vi "DialogRenameVI.vi"(0 "ObjectIn":refnum<class "ClassWriterNative.lvclass">, 1 "ProjectItem":refnum<vi>, 5 "error in (no error)":errorcluster) -> (14 "ObjectOut":refnum<class "ClassWriterNative.lvclass">, 15 "Cancelled":bool, 16 "RenameOption":T1, 19 "error out":errorcluster)   [LabVIEW 2020, in "ClassWriterNative.lvclass"]
uses:
  <resource>/Framework/Providers/Open_GDS/ClassProviders/Provider_LvNativeClass/ClassWriterNative_class/ClassWriterNative.lvclass
  <resource>/Framework/Providers/Open_GDS/ClassProviders/Common/LvIcon_class/GDSLvIcon_ColorControl.ctl
  <resource>/Framework/Providers/Open_GDS/ClassProviders/Provider_BaseClassInterface/ClassWriter_class/RenameViOption.ctl
  <vilib>/Utility/miscctls.llb/LVPoint32TypeDef.ctl
  <vilib>/picture/picture.llb/imagedata.ctl
  <resource>/Framework/Providers/Open_GDS/ClassProviders/Common/LvIcon_class/subvis/GDSLvIcon_TextDataType.ctl
  <resource>/Framework/Providers/Open_GDS/ClassProviders/Common/LvIcon_class/GDSLvIcon_WordCompressionType.ctl
  <resource>/Framework/Providers/Open_GDS/ClassProviders/Common/LvIcon_class/GDSLvIcon_TextAlignment.ctl
  <vilib>/Utility/miscctls.llb/LVPositionTypeDef.ctl
  <vilib>/Utility/miscctls.llb/LVPointTypeDef.ctl
  <resource>/Framework/Providers/Open_GDS/ClassProviders/Provider_BaseClassInterface/ClassWriter_class/ClassWriter.lvclass
panel:
  in  "_ShowContextHelp":bool
  in  "Help":bool
  out "ProductPicture":picture
  out "Ballon":cluster{"Text":string}
  in  "_MethodIcons":bool
  out "_IconPreview":picture caption="Icon Preview"
  in  "_Cancel":bool
  in  "_RenameVI":bool
  out "DragIcon":picture
  in  "FloodFillMask":bool
  in  "_IconSearchText":string caption="Icon search text"
  in  "_Manage":bool
  in  "_Folders":u16(ring) caption="Folders" items=["<All icons>", "...ikael\\Documents\\LabVIEW Data\\Glyphs", "...\\resource\\Framework\\Providers\\Icons", "...Framework\\Providers\\Open_GDS\\Glyphs", "...\\Framework\\Providers\\Open_GDS\\Icons"]
  out "Icons":picture
  in  "_HideHeader":bool=TRUE caption="Force Capital Letters"
  in  "_IconSize":u16(ring) caption="Icon Size" items=["Full", "1 c-term high", "2 c-term high", "3 c-term high"]
  out "Tree":string[](tree)
  in  "_TextAlignment":u16(ring) caption="Text Alignment" items=["Center", "Left", "Right"]
  in  "_MethodIconName":string caption="Body Text"
  in  "_BodyBk":T2 caption="Body Background"
  in  "_BodyText":T2 caption="Body text"
  in  "_FontCompression":enum16{"Auto", "On", "Off"}(ring) caption="Font Compression"
  in  "_CapitalOnly":bool=TRUE caption="Force Capital Letters"
  out "_After":picture caption="New"
  out "_Before":picture caption="Current"
  out "_VIPath":path caption="VI Path"
  in  "NewName":string caption="New Name"
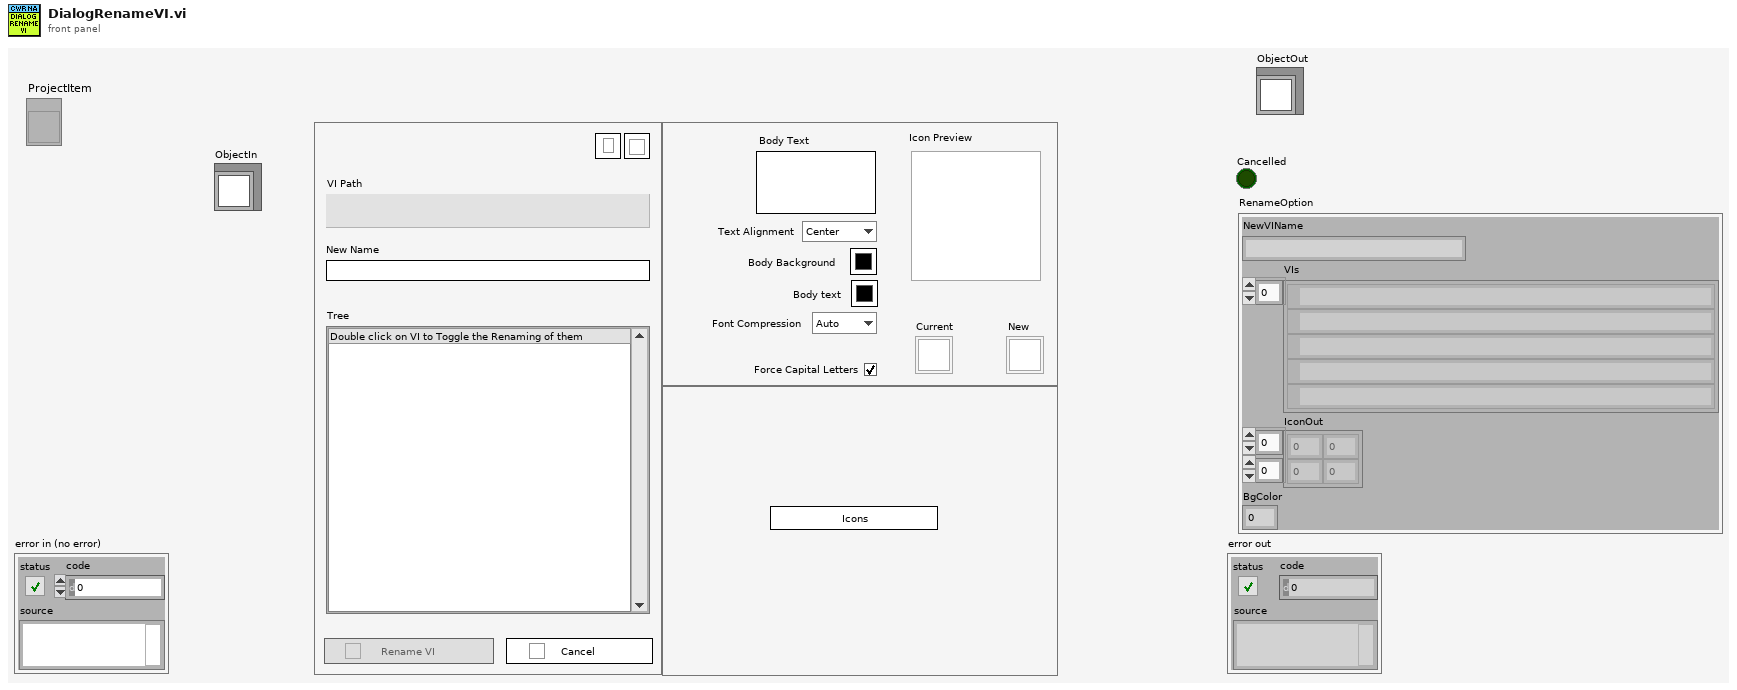
[diagram p1: front panel]
types:
  T1 = typedef "ClassWriter.lvclass/RenameViOption.ctl" = cluster{"NewVIName":string, "VIs":path[], "IconOut":u8[][], "BgColor":u8}
  T2 = typedef "GDSLvIcon_ColorControl.ctl" = cluster{"Decal":bool, "Color":u32}
  T3 = typedef "LVPoint32TypeDef.ctl" = cluster{"Horizontal":i32, "Vertical":i32}
  T4 = typedef "imagedata.ctl" = cluster{"image type":i32, "image depth":i32, "image":u8[], "mask":u8[], "colors":u32[], "Rectangle":cluster{"left":i16, "top":i16, "right":i16, "bottom":i16}}
  T5 = cluster{"ClassIndex":i32, "NewName":string, "Cancelled":bool, "VIref":refnum<vi>, "Class":refnum<vi>, "ClassPath":path, "VIPath":path, "Classes":cluster{i32, refnum<vi>, cluster{"Path":path, "Name":string, "QualifiedName":string}[]}[], "ClassInfos":cluster{"ClassName":string, "ViRelPath":path, "AllVIs":string[], "VI-Path":path, "Private":bool}[], "TreeTags":string[], "Selected":i32[], "CurrentIcon":cluster{"BgIcon":u8[][], "BgIconOffset":cluster{"X":i32, "Y":i32}, "BgIconMask":u8[], "ColorsOkayforiconToBeOnTopOf":u8[]}, "StartIconSize":u16, "Offset":cluster{"X":i32, "Y":i32}, "OldOffset":cluster{"X":i32, "Y":i32}, "ConnectorPaneHeight":i32[], "BodyIcon":u8[][], "Icon exist":bool, "HeaderIcon":u8[][], "BodyIconWidth":i32, "BodyIconHeight":i32, "Frame thickness":i32, "StartRow":i32, "FrameColor":u32, "TextBounds":cluster{"FirstRow":i32, "FirstColumn":i32, "LastRow":i32, "LastColumn":i32}, "Header exists":bool, "HeaderBkColor":u32, "DraggingIcon":bool, "DraggingText":bool, "StartTextDraggingPos":T3, "IconSelected":i32, "BgIconOffset":cluster{"X":i32, "Y":i32}, "IconDropped":i32, "Moving":bool, "Folders":path[], "Icons":T4[], "IconPos":cluster{"left":i16, "top":i16, "right":i16, "bottom":i16}[], "IconPaths":cluster{i32, "path out":path}[], "IconNames":string[], "BgIcon":u8[][], "BgIconMask":u8[], "RenameOption":cluster{"NewVIName":string, "VIs":path[], "IconOut":u8[][], "BgColor":u8}, "StartTime":i32, "FileExtension":string}
  T6 = cluster{"Child Text":string[], "Child Tag":string, "Item Indent":i32, "Child Only?":bool, "Glyph Index":i32}[]
  T7 = cluster{"ClassName":string, "ViRelPath":path, "AllVIs":string[], "VI-Path":path, "Private":bool}
  T8 = enum32{"invalid scope", "public", "private", "protected", "community"}
  T9 = enum8{"Enabled", "Disabled", "Disabled and Grayed Out"}
  T10 = typedef "GDSLvIcon_TextDataType.ctl" = cluster{"Text":string, "Allow Only Capital Chars":bool, "Compression":T11, "Alignment":T12}
  T11 = typedef "GDSLvIcon_WordCompressionType.ctl" = enum16{"Auto", "On", "Off"}
  T12 = typedef "GDSLvIcon_TextAlignment.ctl" = enum16{"Center", "Left", "Right"}
  T13 = typedef "LVPositionTypeDef.ctl" = cluster{"Left":i32, "Top":i32}
  T14 = typedef "LVPointTypeDef.ctl" = cluster{"Horizontal":i16, "Vertical":i16}
  T15 = cluster{"Path":path, "Name":string, "QualifiedName":string}
  T16 = cluster{i32, refnum<vi>, cluster{"Path":path, "Name":string, "QualifiedName":string}[]}
  T17 = cluster{i32, refnum<vi>, cluster{"Path":path, "Name":string, "QualifiedName":string}[]}[]
  T18 = cluster{"Path":path, "Name":string, "QualifiedName":string}[]
  T19 = cluster{"ClassName":string, "ViRelPath":path, "AllVIs":string[], "VI-Path":path, "Private":bool}[]
  T20 = cluster{"BgIcon":u8[][], "BgIconOffset":cluster{"X":i32, "Y":i32}, "BgIconMask":u8[], "ColorsOkayforiconToBeOnTopOf":u8[]}
  T21 = cluster{"FirstRow":i32, "FirstColumn":i32, "LastRow":i32, "LastColumn":i32}
  T22 = typedef "LVBoundsTypeDef.ctl" = cluster{"Width":u32, "Height":u32}
  T23 = cluster{"left":i16, "top":i16, "right":i16, "bottom":i16}[]
  T24 = typedef "eventvkey.ctl" = enum16{"ASCII", "Enter", "Return", "Shift", "Ctrl", "Alt", "Cmd", "Opt", "Caps", "NumLock", "Clear", "Break", "Up", "Down", "Left", "Right", "Insert", "Delete", "Home", "End", "PageUp", "PageDown", "Escape", "Help", "Pause", "ScrollLock", "F1", "F2", "F3", "F4", "F5", "F6", "F7", "F8", "F9", "F10", "F11", "F12", "F13", "F14", "F15", "F16", "F17", "F18", "F19", "F20", "F21", "F22", "F23", "F24", "Play", "VolumeUp", "VolumeDown", "Mute", "Two Byte Char"}
  T25 = cluster{"Shift":bool, "Ctrl":bool, "Alt":bool, "Cmd":bool, "Opt":bool}
  T26 = typedef "LVMouseTypeDef.ctl" = cluster{"Mouse Position":cluster{"X":i32, "Y":i32}, "Mouse Modifiers":cluster{"Button Down":bool, "Shift Mod":bool, "Menu Mod":bool, "Option Mod":bool}}
  T27 = cluster{"left":i16, "top":i16, "right":i16, "bottom":i16}
  T28 = cluster{"NewVIName":string, "VIs":path[], "IconOut":u8[][], "BgColor":u8}
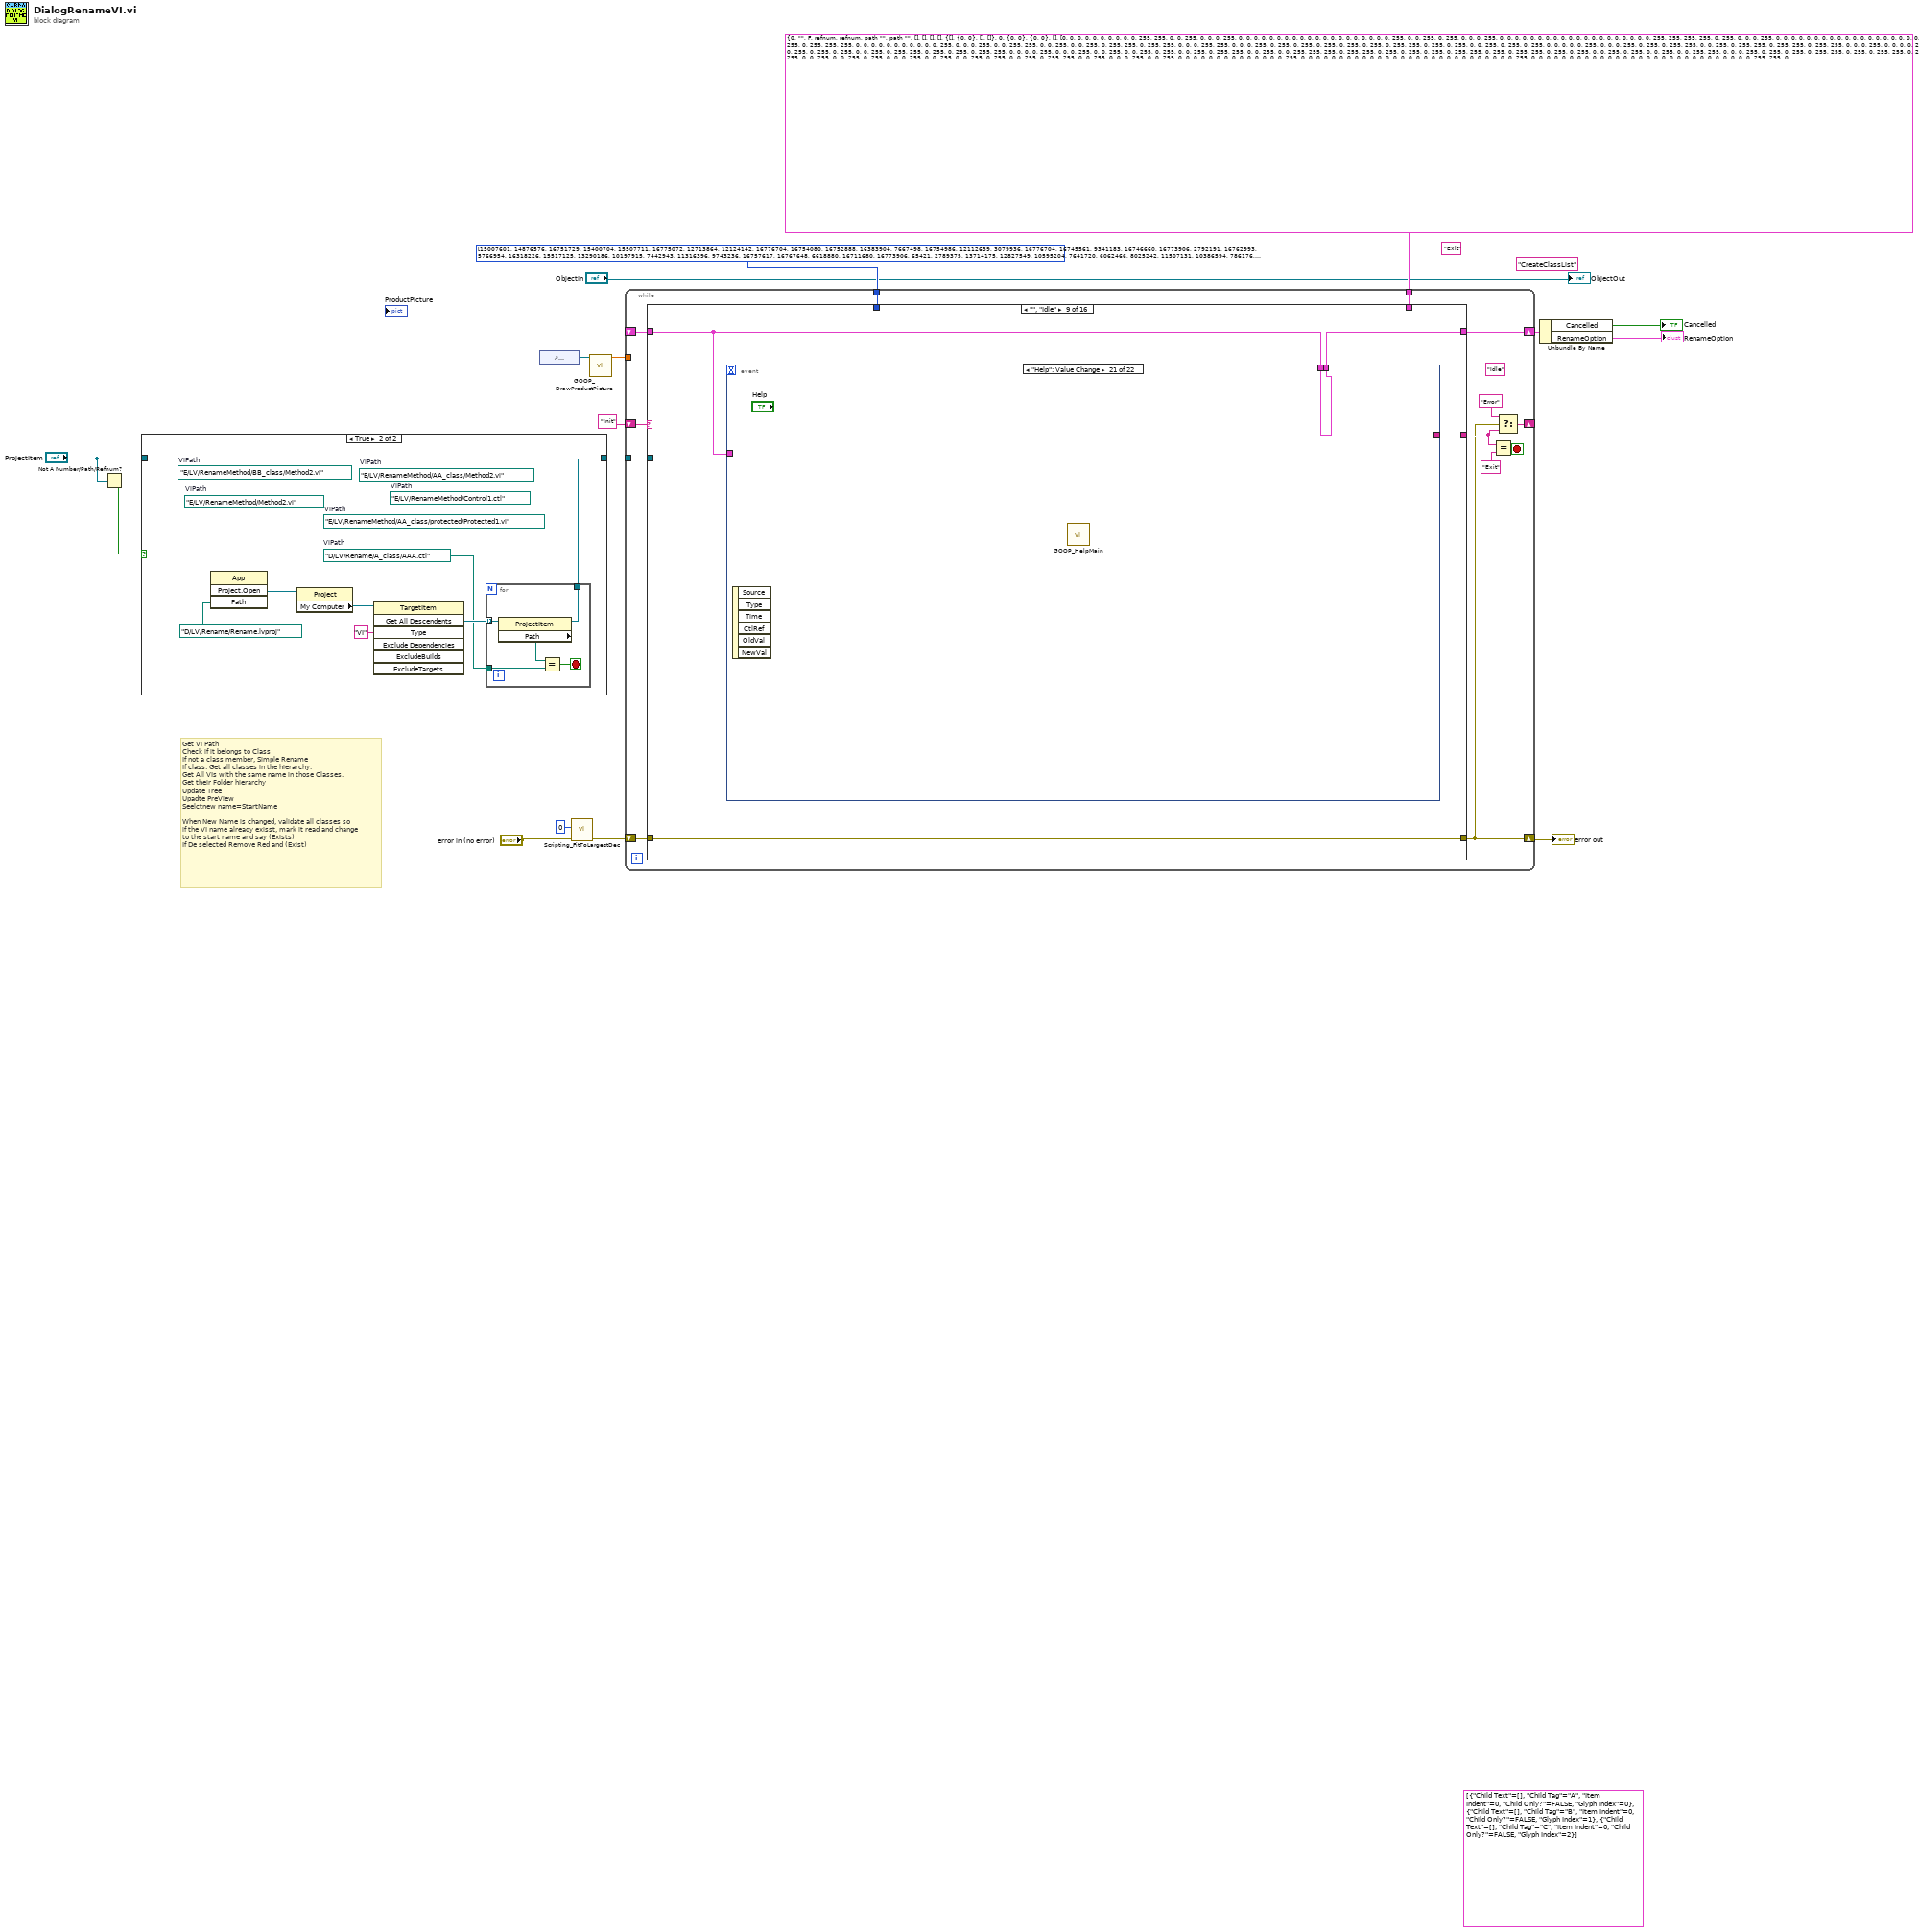
[diagram p0: block diagram]
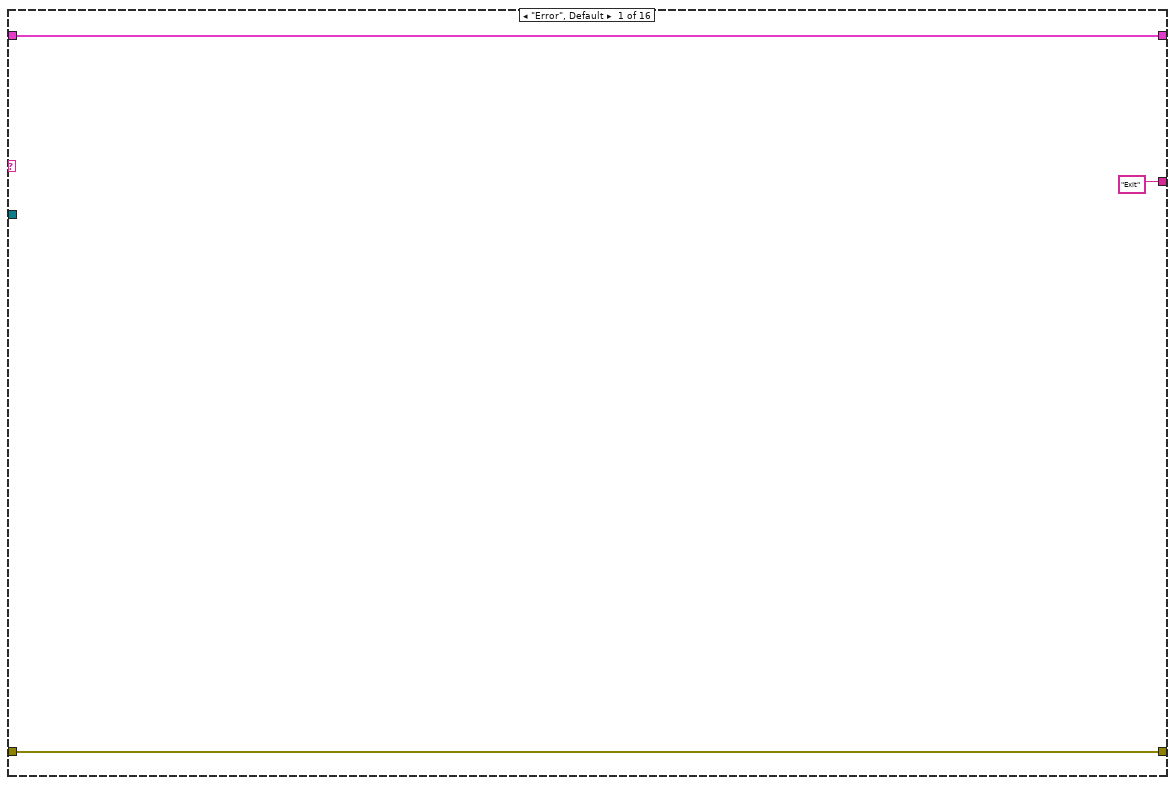
[diagram p3: hidden frame]
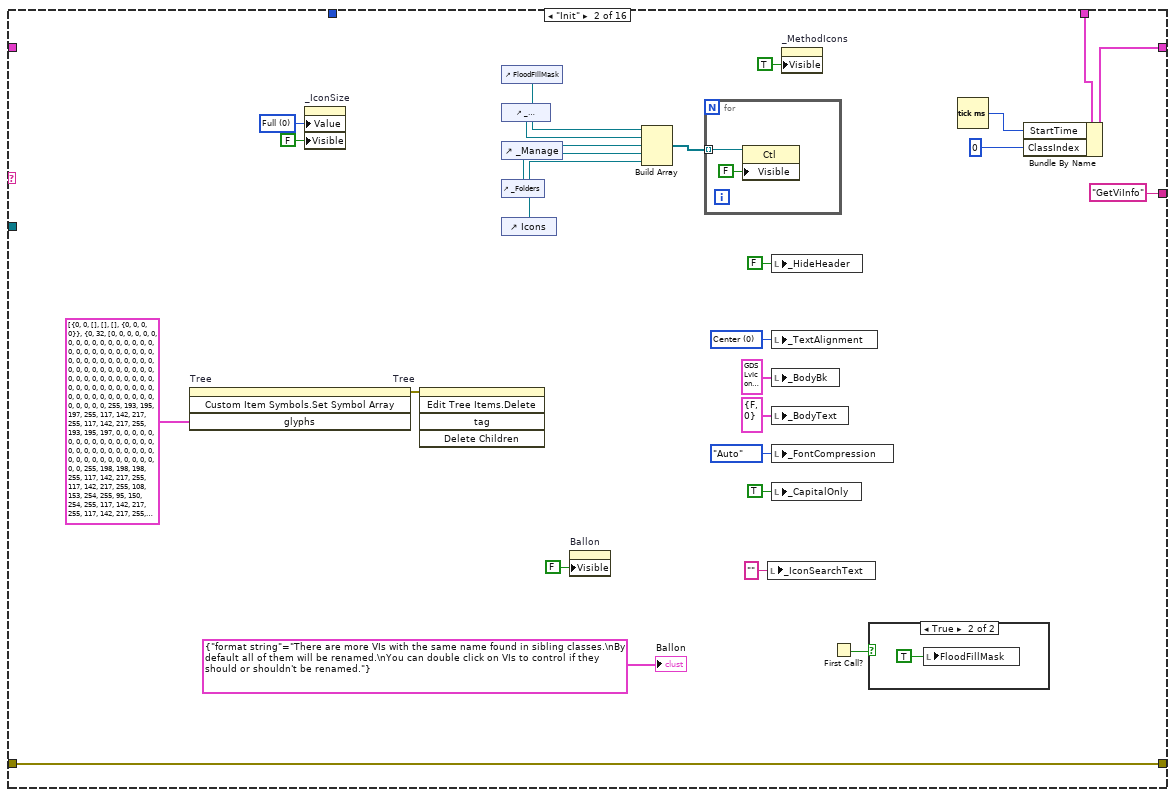
[diagram p4: hidden frame]
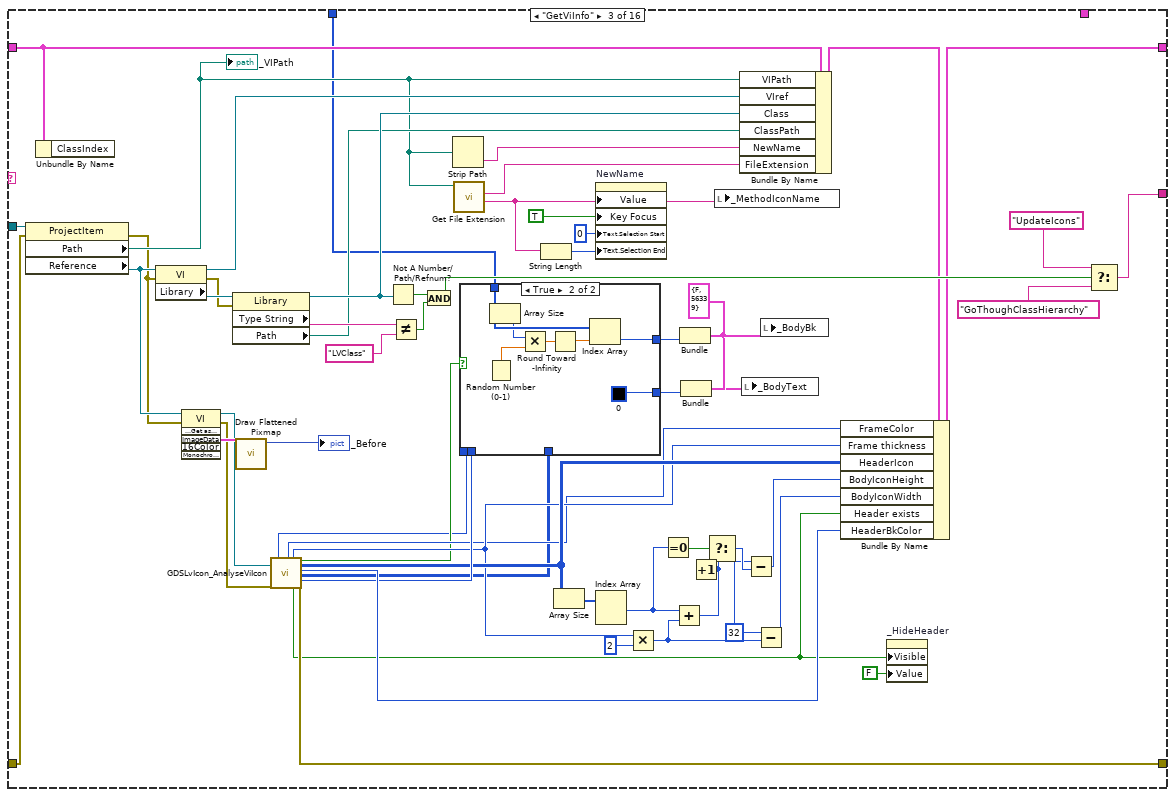
[diagram p6: hidden frame]
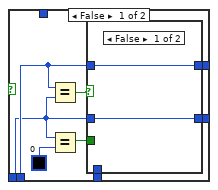
[diagram p7: hidden frame]
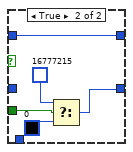
[diagram p8: hidden frame]
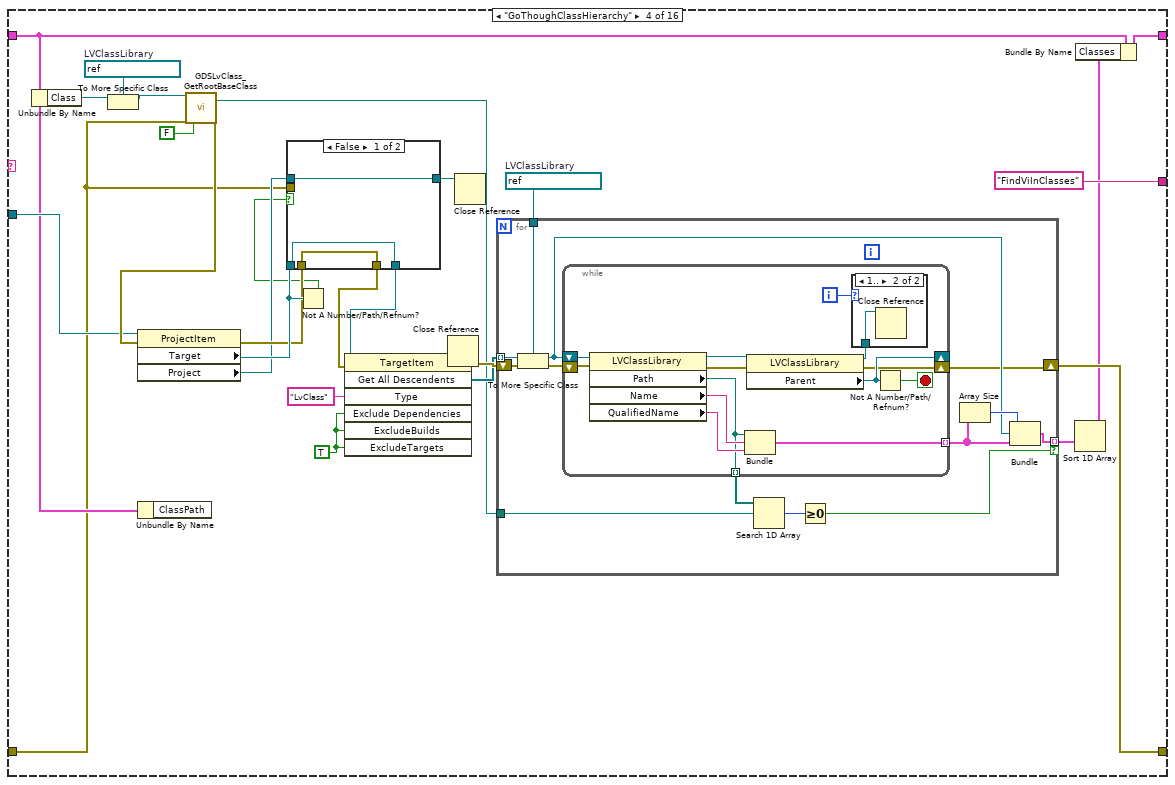
[diagram p9: hidden frame]
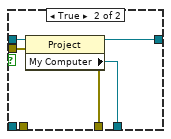
[diagram p10: hidden frame]
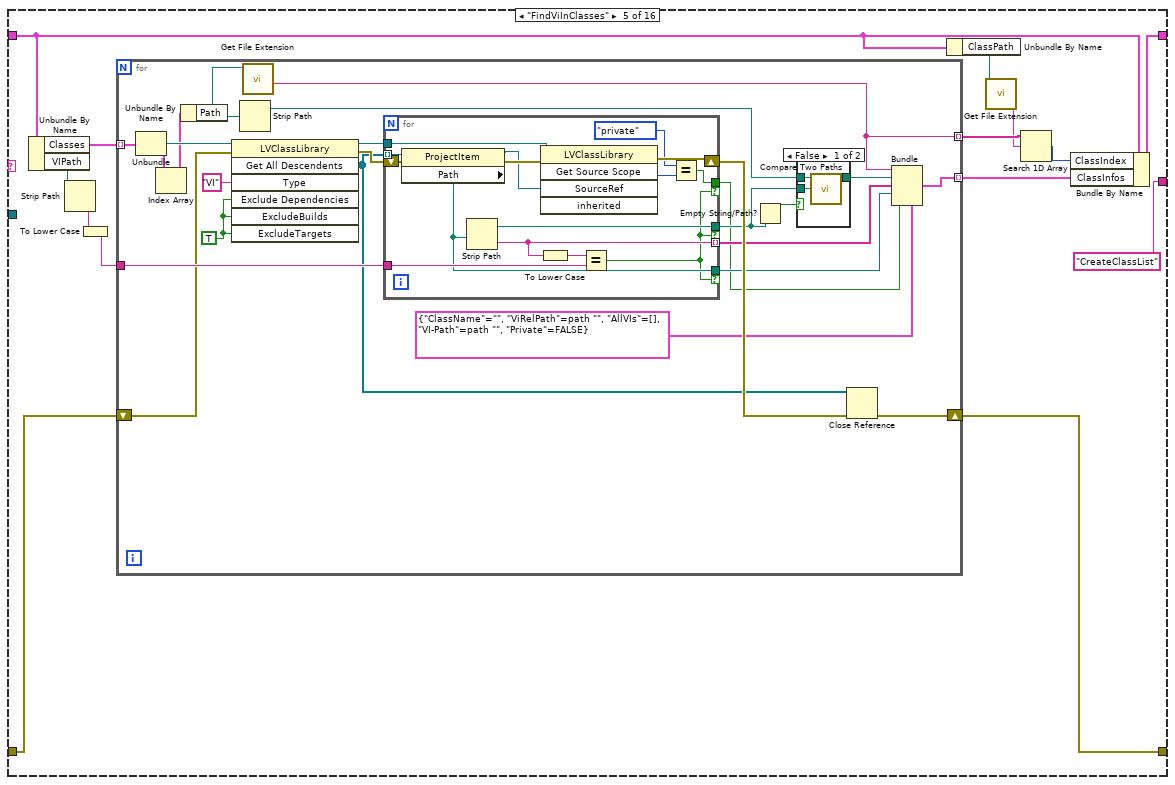
[diagram p12: hidden frame]
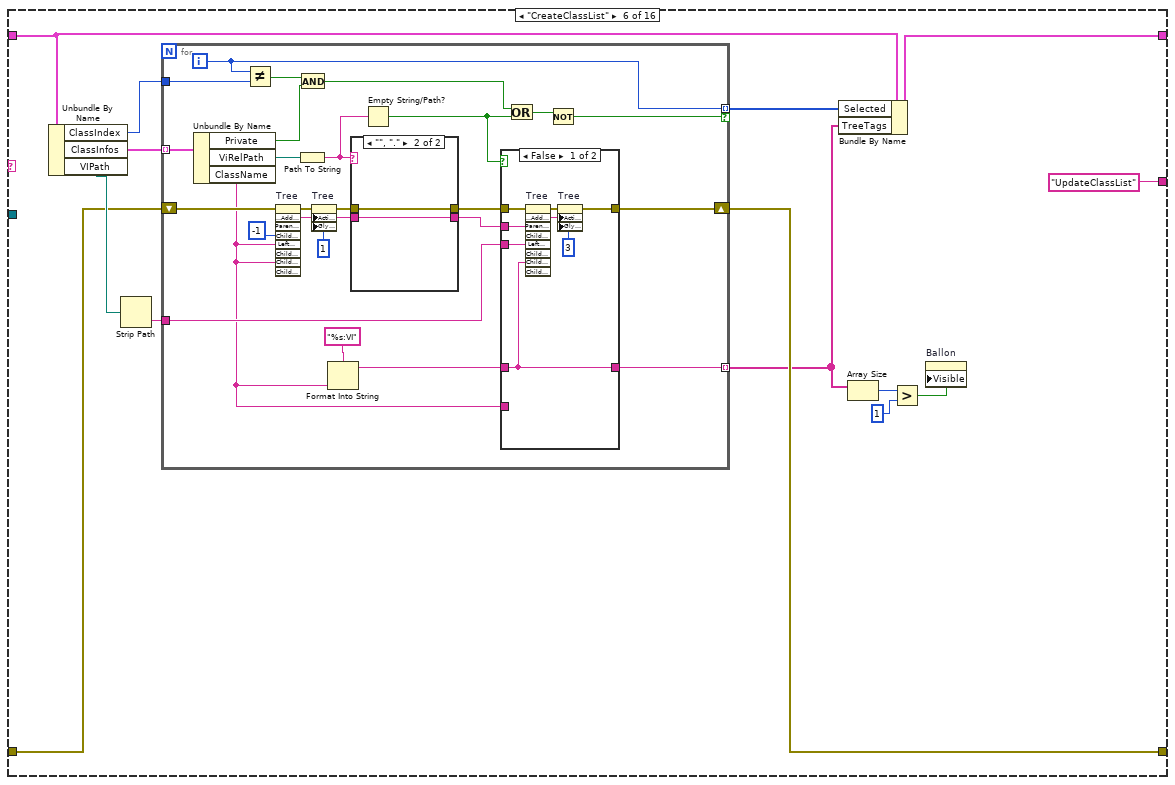
[diagram p14: hidden frame]
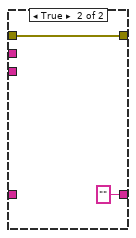
[diagram p15: hidden frame]
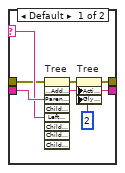
[diagram p16: hidden frame]
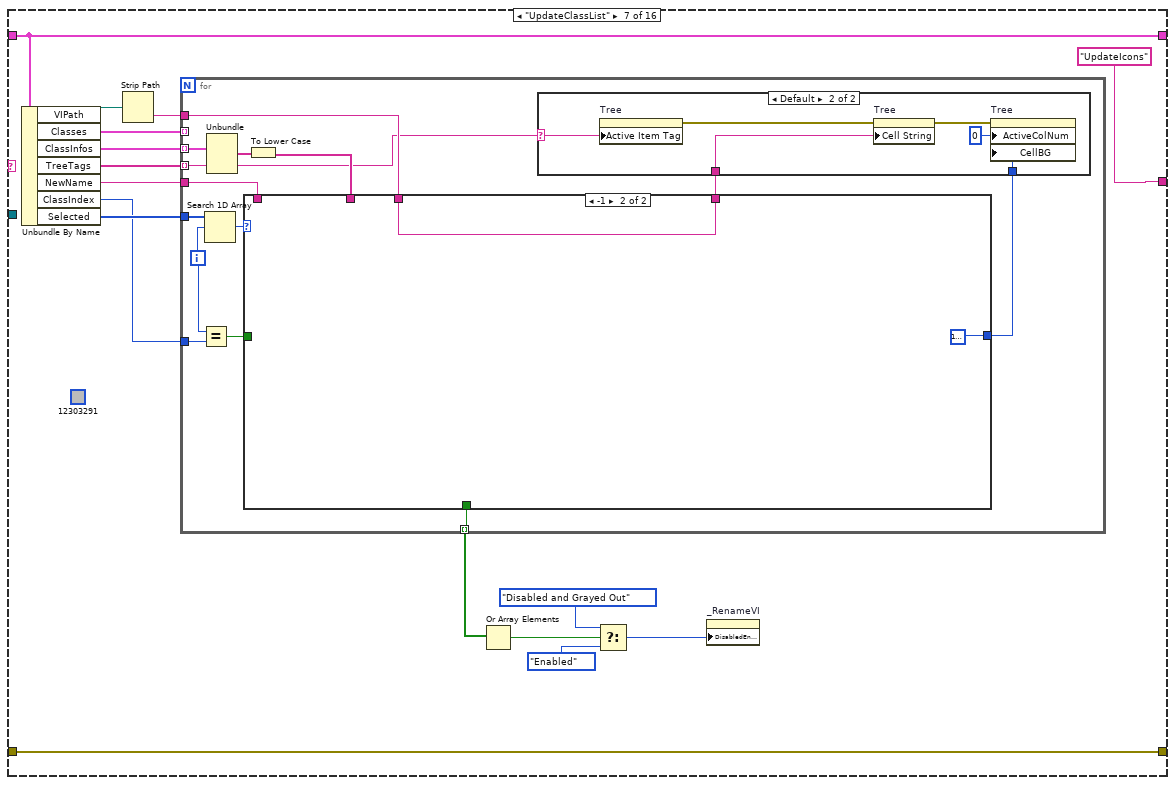
[diagram p17: hidden frame]
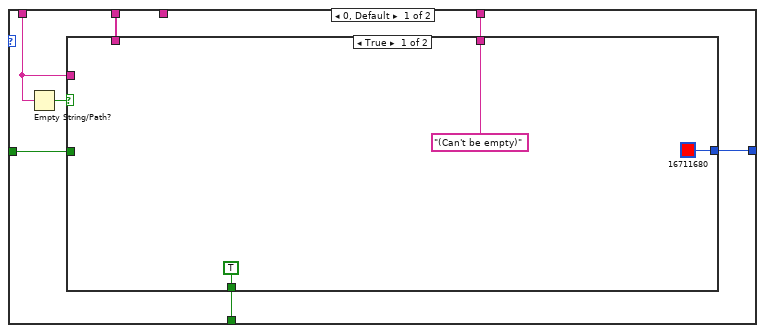
[diagram p19: hidden frame]
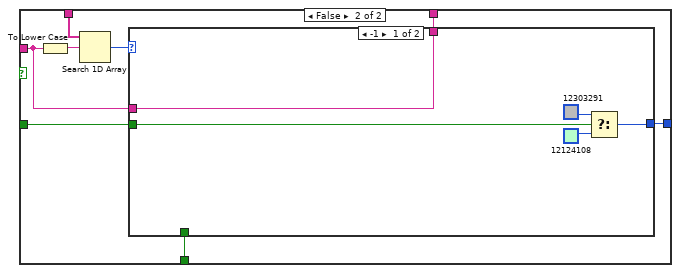
[diagram p20: hidden frame]
diagram:
  (unwired) "CreateClassList"
  (unwired) "Exit"
  (unwired) T6 [{"Child Text"=[], "Child Tag"="A", "Item Indent"=0, "Child Only?"=FALSE, "Glyph Index"=0}, {"Child Text"=[], "Child Tag"="B", "Item Indent"=0, "Child Only?"=FALSE, "Glyph Index"=1}, {"Child Text"=[], "Child Tag"="C", "Item Indent"=0, "Child Only?"=FALSE, "Glyph Index"=2}] ("Items")
  # "Get VI Path\nCheck if it belongs to Class\nIf not a class member, Simple Rename\nIf class: Get all classes in the hierarchy.\nGet All VIs with the same name in those Classes.\nGet their Folder hierarchy\nUpdate Tree\nUpadte PreView\nSeelctnew name=StartName\n\nWhen New Name is changed, validate all classes so\nif the VI name already exisst, mark it read and change\nto the start name and say (Exists)\nIf De selected Remove Red and (Exist)"
  n1 = Not A Number/Path/Refnum?(number/path/refnum="ProjectItem") -> (NaN/Path/Refnum?=w12:bool)
  n2 = case shown="True" w12 {
    tunnel: "ProjectItem" -> [w17 _]
    tunnel: [w17 w19] -> w6
    frame False {
    }
    frame True {
      (unwired) path "E:/LV/RenameMethod/Control1.ctl"  # ViPath
      (unwired) path "E:/LV/RenameMethod/Method2.vi"  # ViPath
      (unwired) path "E:/LV/RenameMethod/BB_class/Method2.vi"  # ViPath
      (unwired) path "E:/LV/RenameMethod/AA_class/Method2.vi"  # ViPath
      (unwired) path "E:/LV/RenameMethod/AA_class/protected/Protected1.vi"  # ViPath
      w18 = path "D:/LV/Rename/A_class/AAA.ctl"  # ViPath
      n3 = invoke class="App" method="Project.Open"("Path"=path "D:/LV/Rename/Rename.lvproj") -> ("Project:Open"=w23:refnum<vi>)  [unwired: 3 in, 3 out]
      n4 = property class="Project"(reference=w23) -> ("My Computer"=w22:refnum<vi>)  [unwired: 1 in, 2 out]
      n5 = invoke class="TargetItem" method="Get All Descendents"(reference=w22, "Type"="VI") -> ("All Descendents"=w20:refnum<vi>[])  [unwired: 5 in, 6 out]
      n6 = for {
        tunnel: w20 -> [w29] mode=indexing
        tunnel: w18 -> [w27]
        tunnel: [w25] -> w19
        stop <- w26 stop-if-true
        n7 = property class="ProjectItem"(reference=w29) -> (reference out=w25:refnum<vi>, "Path"=w28:path)  [unwired: 1 in, 1 out]
        n8 = Equal?(x=w28, y=w27) -> (x = y?=w26:bool)
      }
    }
  }
  n9 = control-ref of="ProductPicture"() -> (w4:refnum<vi>)
  n10 = call <resource>:"Scripting_FitToLargestDec.vi"("error in (no error)"="error in (no error)", "border spacing (2 px)"=0) -> ("error out"=w1:errorcluster)  [unwired: 4 in, 1 out]
  n11 = call <resource>:"GOOP_DrawProductPicture.vi"("ProductPictureControl"=w4) -> ("Zoom Factor"=w5:sgl)  [unwired: 10 in]
  n12 = while {
    shift-right: [w35] -> w14
    shift-left: w1 -> [w42]
    shift-right: [w40] -> _
    shift-left: "Init" -> [w41]
    shift-right: [w31] -> w16
    shift-left: _ -> [w34]
    tunnel: w6 -> [w33]
    tunnel: T5 {"ClassIndex"=0, "NewName"="", "Cancelled"=FALSE, "VIref"=refnum, "Class"=refnum, "ClassPath"=path "", "VIPath"=path "", "Classes"=[], "ClassInfos"=[], "TreeTags"=[], "Selected"=[], "CurrentIcon"={"BgIcon"=[], "BgIconOffset"={"X"=0, "Y"=0}, "BgIconMask"=[], "ColorsOkayforiconToBeOnTopOf"=[]}, "StartIconSize"=0, "Offset"={"X"=0, "Y"=0}, "OldOffset"={"X"=0, "Y"=0}, "ConnectorPaneHeight"=[], "BodyIcon"=[[0, 0, 0, 0, 0, 0, 0, 0, 0, 0, 255, 255, 0, 0, 255, 0, 0, 0, 255, 0, 0, 0, 0, 0, 0, 0, 0, 0, 0, 0], [0, 0, 0, 0, 0, 0, 0, 0, 0, 255, 0, 0, 255, 0, 255, 0, 0, 0, 255, 0, 0, 0, 0, 0, 0, 0, 0, 0, 0, 0], [0, 0, 0, 0, 0, 0, 0, 0, 0, 255, 255, 255, 255, 0, 255, 0, 0, 0, 255, 0, 0, 0, 0, 0, 0, 0, 0, 0, 0, 0], [0, 0, 0, 0, 0, 0, 0, 0, 0, 255, 0, 0, 255, 0, 255, 0, 0, 0, 255, 0, 0, 0, 0, 0, 0, 0, 0, 0, 0, 0], [0, 0, 0, 0, 0, 0, 0, 0, 0, 255, 0, 0, 255, 0, 255, 255, 255, 0, 255, 255, 255, 0, 0, 0, 0, 0, 0, 0, 0, 0], [0, 0, 255, 0, 0, 0, 255, 0, 0, 255, 255, 0, 0, 255, 0, 0, 255, 0, 255, 255, 0, 255, 255, 0, 0, 0, 255, 255, 0, 0], [0, 255, 0, 255, 0, 255, 0, 255, 0, 255, 0, 255, 0, 255, 255, 0, 255, 0, 255, 0, 0, 255, 0, 255, 0, 255, 0, 0, 0, 0], [0, 255, 0, 0, 0, 255, 0, 255, 0, 255, 255, 0, 0, 255, 0, 255, 255, 0, 255, 255, 0, 255, 255, 0, 0, 0, 255, 0, 0, 0], [0, 255, 0, 255, 0, 255, 0, 255, 0, 255, 0, 255, 0, 255, 0, 0, 255, 0, 255, 0, 0, 255, 0, 255, 0, 0, 0, 255, 0, 0], [0, 0, 255, 0, 0, 0, 255, 0, 0, 255, 0, 255, 0, 255, 0, 0, 255, 0, 255, 255, 0, 255, 0, 255, 0, 255, 255, 0, 0, 0], [0, 255, 0, 0, 0, 255, 0, 0, 255, 0, 0, 255, 0, 255, 0, 0, 255, 0, 255, 255, 0, 0, 255, 0, 0, 255, 255, 255, 0, 255], [255, 0, 255, 0, 255, 0, 255, 0, 255, 255, 0, 255, 0, 255, 255, 0, 255, 0, 255, 0, 0, 255, 0, 255, 0, 0, 255, 0, 0, 255], [255, 0, 0, 0, 255, 0, 255, 0, 255, 0, 255, 255, 0, 255, 0, 255, 255, 0, 255, 255, 0, 255, 0, 0, 0, 0, 255, 0, 0, 255], [255, 0, 255, 0, 255, 0, 255, 0, 255, 0, 0, 255, 0, 255, 0, 0, 255, 0, 255, 0, 0, 255, 0, 255, 0, 0, 255, 0, 0, 255], [0, 255, 0, 0, 0, 255, 0, 0, 255, 0, 0, 255, 0, 255, 0, 0, 255, 0, 255, 255, 0, 0, 255, 0, 0, 0, 255, 0, 0, 255], [0, 0, 0, 0, 0, 0, 0, 0, 0, 0, 0, 0, 0, 0, 255, 0, 0, 0, 0, 0, 0, 0, 0, 0, 0, 0, 0, 0, 0, 0], [0, 0, 0, 0, 0, 0, 0, 0, 0, 0, 0, 0, 0, 255, 0, 0, 0, 0, 0, 0, 0, 0, 0, 0, 0, 0, 0, 0, 0, 0], [0, 0, 0, 0, 0, 0, 0, 0, 0, 0, 0, 0, 0, 255, 255, 0, 0, 0, 0, 0, 0, 0, 0, 0, 0, 0, 0, 0, 0, 0], [0, 0, 0, 0, 0, 0, 0, 0, 0, 0, 0, 0, 0, 255, 0, 255, 0, 0, 0, 0, 0, 0, 0, 0, 0, 0, 0, 0, 0, 0], [0, 0, 0, 0, 0, 0, 0, 0, 0, 0, 0, 0, 0, 0, 255, 0, 0, 0, 0, 0, 0, 0, 0, 0, 0, 0, 0, 0, 0, 0], [0, 0, 0, 0, 0, 0, 0, 0, 0, 0, 0, 0, 0, 0, 0, 0, 0, 0, 0, 0, 0, 0, 0, 0, 0, 0, 0, 0, 0, 0], [0, 0, 0, 0, 0, 0, 0, 0, 0, 0, 0, 0, 0, 0, 0, 0, 0, 0, 0, 0, 0, 0, 0, 0, 0, 0, 0, 0, 0, 0]], "Icon exist"=FALSE, "HeaderIcon"=[], "BodyIconWidth"=0, "BodyIconHeight"=0, "Frame thickness"=3, "StartRow"=0, "FrameColor"=0, "TextBounds"={"FirstRow"=2, "FirstColumn"=1, "LastRow"=6, "LastColumn"=27}, "Header exists"=FALSE, "HeaderBkColor"=0, "DraggingIcon"=FALSE, "DraggingText"=FALSE, "StartTextDraggingPos"={"Horizontal"=0, "Vertical"=0}, "IconSelected"=0, "BgIconOffset"={"X"=0, "Y"=0}, "IconDropped"=-1, "Moving"=FALSE, "Folders"=[], "Icons"=[], "IconPos"=[], "IconPaths"=[], "IconNames"=[], "BgIcon"=[], "BgIconMask"=[], "RenameOption"={"NewVIName"="", "VIs"=[], "IconOut"=[], "BgColor"=0}, "StartTime"=0, "FileExtension"=""} -> [w32]
    tunnel: u32[] [15007601, 14876576, 16751729, 15400704, 15507711, 16775072, 12713864, 12124142, 16776704, 16754080, 16752888, 16383904, 7667498, 16754986, 12112639, 3079936, 16776704, 16745561, 9341183, 16746660, 16773906, 2792191, 16762993, 5766954, 16318226, 15517125, 13290186, 10197915, 7442943, 11316396, 9743236, 16757617, 16767648, 6618880, 16711680, 16773906, 65421, 2789375, 13714175, 12827549, 10595204, 7641720, 6062466, 8025242, 11507131, 10386594, 786176, 8584960, 16318208, 16731648, 16755616, 16734715, 14399157, 16754801, 16714752, 10026888, 3524608] -> [w30]
    tunnel: w5 -> [_]
    stop <- w39 stop-if-true
    (unwired) "Idle"
    n13 = case shown="\"\", \"Idle\"" w41 {
      selector: w41 -> [_ _ _ _ _ _ _ _ _ _ w816 _ _ w993 _ w1145]
      tunnel: w42 -> [w45 w71 w102 w159 w229 w285 w349 w447 w459 w810 w858 w865 w950 w1000 w1128 w1149]
      tunnel: [w45 w71 w104 w158 w228 w284 w349 w411 w459 w810 w858 w864 w949 w999 w1128 w1148] -> w35
      tunnel: ["Exit" "GetViInfo" w130 "FindViInClasses" "CreateClassList" "UpdateClassList" "UpdateIcons" "Idle" w460 "UpdateIcon" ("y") w815 "ReadIcons" "DrawIcons" ("y") "Idle" ("y") "Generate icon" w1147] -> w36
      tunnel: w34 -> [w43 _ w134 w165 w223 w289 w348 w401 w458 w801 w817 w862 w953 w998 w1121 w1135]
      tunnel: w33 -> [_ _ w133 w166 _ _ _ _ _ _ _ _ _ _ _ _]
      tunnel: w32 -> [_ w68 _ _ _ _ _ _ _ _ _ _ _ _ _ _]
      tunnel: [w43 w70 w92 w162 w227 w282 w348 w418 w461 w800 w817 w861 w952 w997 w1120 w1144] -> w31
      tunnel: w30 -> [_ _ w80 _ _ _ _ _ _ _ _ _ _ _ _ _]
      frame "Error", Default {
      }
      frame "Init" {
        w62 = u16 0 items=["Center", "Left", "Right"] ("_TextAlignment")
        w64 = u16 0 items=["Full", "1 c-term high", "2 c-term high", "3 c-term high"] ("_IconSize")
        n14 = invoke on="Tree" class="Tree (strict)" method="Custom Item Symbols.Set Symbol Array"("glyphs"=T4[] [{"image type"=0, "image depth"=0, "image"=[], "mask"=[], "colors"=[], "Rectangle"={"left"=0, "top"=0, "right"=0, "bottom"=0}}, {"image type"=0, "image depth"=32, "image"=[0, 0, 0, 0, 0, 0, 0, 0, 0, 0, 0, 0, 0, 0, 0, 0, 0, 0, 0, 0, 0, 0, 0, 0, 0, 0, 0, 0, 0, 0, 0, 0, 0, 0, 0, 0, 0, 0, 0, 0, 0, 0, 0, 0, 0, 0, 0, 0, 0, 0, 0, 0, 0, 0, 0, 0, 0, 0, 0, 0, 0, 0, 0, 0, 0, 0, 0, 0, 0, 0, 0, 0, 0, 0, 0, 0, 0, 0, 0, 0, 0, 0, 0, 0, 0, 0, 0, 0, 255, 193, 195, 197, 255, 117, 142, 217, 255, 117, 142, 217, 255, 193, 195, 197, 0, 0, 0, 0, 0, 0, 0, 0, 0, 0, 0, 0, 0, 0, 0, 0, 0, 0, 0, 0, 0, 0, 0, 0, 0, 0, 0, 0, 0, 0, 0, 0, 0, 0, 0, 0, 0, 0, 0, 0, 255, 198, 198, 198, 255, 117, 142, 217, 255, 117, 142, 217, 255, 108, 153, 254, 255, 95, 150, 254, 255, 117, 142, 217, 255, 117, 142, 217, 255, 193, 195, 197, 0, 0, 0, 0, 0, 0, 0, 0, 0, 0, 0, 0, 0, 0, 0, 0, 0, 0, 0, 0, 0, 0, 0, 0, 255, 198, 198, 198, 255, 117, 142, 217, 255, 117, 142, 217, 255, 108, 153, 254, 255, 108, 153, 254, 255, 127, 159, 255, 255, 127, 159, 255, 255, 95, 150, 254, 255, 95, 150, 254, 255, 117, 142, 217, 255, 117, 142, 217, 255, 191, 194, 197, 0, 0, 0, 0, 0, 0, 0, 0, 0, 0, 0, 0, 0, 0, 0, 0, 255, 38, 82, 217, 255, 102, 152, 254, 255, 115, 150, 254, 255, 127, 159, 255, 255, 127, 159, 255, 255, 127, 159, 255, 255, 127, 159, 255, 255, 127, 159, 255, 255, 127, 159, 255, 255, 98, 137, 254, 255, 83, 146, 254, 255, 18, 18, 118, 0, 0, 0, 0, 0, 0, 0, 0, 0, 0, 0, 0, 0, 0, 0, 0, 255, 25, 82, 255, 255, 61, 84, 234, 255, 116, 137, 243, 255, 127, 159, 255, 255, 127, 159, 255, 255, 127, 159, 255, 255, 96, 146, 254, 255, 96, 146, 254, 255, 96, 146, 254, 255, 11, 12, 134, 255, 11, 11, 134, 255, 0, 0, 128, 0, 0, 0, 0, 0, 0, 0, 0, 0, 0, 0, 0, 0, 0, 0, 0, 255, 25, 82, 255, 255, 25, 82, 255, 255, 25, 82, 255, 255, 50, 81, 238, 255, 50, 81, 238, 255, 127, 159, 255, 255, 96, 146, 254, 255, 11, 12, 134, 255, 11, 12, 134, 255, 0, 0, 128, 255, 0, 0, 128, 255, 8, 8, 107, 0, 0, 0, 0, 0, 0, 0, 0, 0, 0, 0, 0, 0, 0, 0, 0, 255, 25, 82, 255, 255, 25, 82, 255, 255, 25, 82, 255, 255, 50, 81, 238, 255, 50, 81, 238, 255, 50, 81, 238, 255, 11, 12, 134, 255, 11, 12, 134, 255, 11, 12, 134, 255, 0, 0, 128, 255, 11, 11, 134, 255, 8, 8, 107, 0, 0, 0, 0, 0, 0, 0, 0, 0, 0, 0, 0, 0, 0, 0, 0, 255, 25, 82, 255, 255, 25, 82, 255, 255, 25, 82, 255, 255, 50, 81, 238, 255, 50, 81, 238, 255, 50, 81, 238, 255, 11, 12, 134, 255, 11, 12, 134, 255, 11, 12, 134, 255, 0, 0, 128, 255, 11, 11, 134, 255, 8, 8, 107, 0, 0, 0, 0, 0, 0, 0, 0, 0, 0, 0, 0, 0, 0, 0, 0, 255, 25, 82, 255, 255, 25, 82, 255, 255, 25, 82, 255, 255, 50, 81, 238, 255, 50, 81, 238, 255, 50, 81, 238, 255, 11, 12, 134, 255, 11, 12, 134, 255, 11, 12, 134, 255, 0, 0, 128, 255, 11, 11, 134, 255, 8, 8, 107, 0, 0, 0, 0, 0, 0, 0, 0, 0, 0, 0, 0, 0, 0, 0, 0, 255, 25, 82, 255, 255, 25, 82, 255, 255, 25, 82, 255, 255, 50, 81, 238, 255, 50, 81, 238, 255, 50, 81, 238, 255, 11, 12, 134, 255, 11, 12, 134, 255, 11, 12, 134, 255, 0, 0, 128, 255, 11, 11, 134, 255, 8, 8, 107, 0, 0, 0, 0, 0, 0, 0, 0, 0, 0, 0, 0, 0, 0, 0, 0, 255, 48, 92, 227, 255, 33, 81, 249, 255, 25, 82, 255, 255, 48, 77, 237, 255, 48, 77, 237, 255, 48, 77, 237, 255, 0, 0, 128, 255, 0, 0, 128, 255, 0, 0, 128, 255, 11, 11, 134, 255, 11, 11, 134, 255, 35, 36, 108, 0, 0, 0, 0, 0, 0, 0, 0, 0, 0, 0, 0, 0, 0, 0, 0, 255, 190, 193, 197, 255, 37, 82, 217, 255, 37, 82, 217, 255, 58, 80, 232, 255, 58, 80, 232, 255, 48, 77, 237, 255, 0, 0, 128, 255, 11, 11, 134, 255, 11, 11, 134, 255, 35, 36, 108, 255, 35, 36, 108, 255, 182, 188, 196, 0, 0, 0, 0, 0, 0, 0, 0, 0, 0, 0, 0, 0, 0, 0, 0, 0, 0, 0, 0, 0, 0, 0, 0, 255, 186, 190, 196, 255, 49, 82, 179, 255, 49, 82, 179, 255, 58, 80, 232, 255, 11, 11, 134, 255, 35, 36, 108, 255, 35, 36, 108, 255, 182, 188, 196, 0, 0, 0, 0, 0, 0, 0, 0, 0, 0, 0, 0, 0, 0, 0, 0, 0, 0, 0, 0, 0, 0, 0, 0, 0, 0, 0, 0, 0, 0, 0, 0, 0, 0, 0, 0, 0, 0, 0, 0, 255, 193, 195, 197, 255, 49, 82, 179, 255, 35, 36, 108, 255, 182, 188, 196, 0, 0, 0, 0, 0, 0, 0, 0, 0, 0, 0, 0, 0, 0, 0, 0, 0, 0, 0, 0, 0, 0, 0, 0, 0, 0, 0, 0, 0, 0, 0, 0, 0, 0, 0, 0, 0, 0, 0, 0, 0, 0, 0, 0, 0, 0, 0, 0, 0, 0, 0, 0, 0, 0, 0, 0, 0, 0, 0, 0, 0, 0, 0, 0, 0, 0, 0, 0, 0, 0, 0, 0, 0, 0, 0, 0, 0, 0, 0, 0, 0, 0, 0, 0, 0, 0, 0, 0], "mask"=[0, 0, 3, 192, 15, 240, 63, 252, 63, 252, 63, 252, 63, 252, 63, 252, 63, 252, 63, 252, 63, 252, 63, 252, 63, 252, 15, 240, 3, 192, 0, 0], "colors"=[], "Rectangle"={"left"=0, "top"=0, "right"=16, "bottom"=16}}, {"image type"=0, "image depth"=32, "image"=[0, 0, 0, 0, 0, 0, 0, 0, 0, 0, 0, 0, 1, 64, 64, 64, 1, 64, 64, 64, 1, 64, 64, 64, 1, 64, 64, 64, 0, 0, 0, 0, 2, 64, 64, 64, 4, 64, 64, 64, 5, 64, 64, 64, 4, 64, 64, 64, 4, 64, 64, 64, 3, 64, 64, 64, 2, 64, 64, 64, 0, 0, 0, 0, 2, 64, 64, 64, 4, 64, 64, 64, 33, 122, 122, 122, 97, 133, 133, 133, 71, 127, 127, 127, 15, 64, 64, 64, 11, 64, 64, 64, 18, 102, 102, 102, 113, 131, 131, 131, 184, 132, 132, 132, 242, 130, 130, 130, 155, 142, 142, 142, 163, 141, 141, 141, 200, 155, 155, 155, 54, 106, 106, 106, 0, 0, 0, 0, 103, 136, 136, 136, 201, 138, 138, 138, 243, 139, 139, 139, 255, 140, 140, 140, 199, 133, 133, 133, 133, 120, 120, 120, 188, 130, 130, 130, 229, 131, 131, 131, 255, 146, 146, 146, 255, 150, 150, 150, 255, 156, 156, 156, 242, 181, 181, 181, 242, 211, 211, 211, 255, 253, 253, 253, 180, 93, 93, 93, 0, 0, 0, 0, 226, 139, 139, 139, 255, 140, 140, 140, 255, 138, 138, 138, 255, 134, 134, 134, 255, 137, 137, 137, 255, 147, 147, 147, 255, 155, 155, 155, 255, 151, 151, 151, 255, 200, 200, 200, 255, 235, 235, 235, 255, 246, 246, 246, 255, 238, 238, 238, 255, 233, 233, 233, 255, 228, 228, 228, 186, 50, 50, 50, 0, 0, 0, 0, 230, 139, 139, 139, 255, 140, 140, 140, 255, 148, 148, 148, 255, 158, 158, 158, 255, 162, 162, 162, 255, 192, 192, 192, 255, 217, 217, 217, 255, 247, 247, 247, 255, 236, 236, 236, 255, 230, 230, 230, 255, 225, 225, 225, 255, 222, 222, 222, 255, 226, 226, 226, 251, 173, 173, 173, 181, 47, 47, 47, 0, 0, 0, 0, 247, 144, 144, 144, 255, 141, 141, 141, 255, 173, 173, 173, 255, 244, 244, 244, 255, 245, 245, 245, 255, 238, 238, 238, 255, 231, 231, 231, 255, 227, 227, 227, 255, 221, 221, 221, 255, 217, 217, 217, 255, 213, 213, 213, 255, 210, 210, 210, 255, 219, 219, 219, 238, 106, 106, 106, 169, 61, 61, 61, 0, 0, 0, 0, 230, 138, 138, 138, 255, 137, 137, 137, 255, 209, 209, 209, 255, 236, 236, 236, 255, 228, 228, 228, 255, 224, 224, 224, 255, 220, 220, 220, 255, 217, 217, 217, 255, 210, 210, 210, 255, 206, 206, 206, 255, 202, 202, 202, 255, 199, 199, 199, 255, 203, 203, 203, 217, 59, 59, 59, 149, 64, 64, 64, 0, 0, 0, 0, 230, 136, 136, 136, 255, 147, 147, 147, 255, 218, 218, 218, 255, 221, 221, 221, 255, 216, 216, 216, 255, 212, 212, 212, 255, 208, 208, 208, 255, 205, 205, 205, 255, 198, 198, 198, 255, 195, 195, 195, 255, 191, 191, 191, 255, 191, 191, 191, 255, 170, 170, 170, 189, 42, 42, 42, 123, 64, 64, 64, 0, 0, 0, 0, 230, 134, 134, 134, 255, 165, 165, 165, 255, 213, 213, 213, 255, 206, 206, 206, 255, 203, 203, 203, 255, 199, 199, 199, 255, 195, 195, 195, 255, 192, 192, 192, 255, 185, 185, 185, 255, 181, 181, 181, 255, 177, 177, 177, 255, 183, 183, 183, 244, 112, 112, 112, 153, 54, 54, 54, 92, 64, 64, 64, 0, 0, 0, 0, 230, 135, 135, 135, 255, 177, 177, 177, 255, 202, 202, 202, 255, 195, 195, 195, 255, 192, 192, 192, 255, 188, 188, 188, 255, 184, 184, 184, 255, 180, 180, 180, 255, 174, 174, 174, 255, 170, 170, 170, 255, 166, 166, 166, 255, 172, 172, 172, 225, 66, 66, 66, 124, 64, 64, 64, 63, 64, 64, 64, 0, 0, 0, 0, 230, 139, 139, 139, 255, 183, 183, 183, 255, 189, 189, 189, 255, 184, 184, 184, 255, 181, 181, 181, 255, 177, 177, 177, 255, 173, 173, 173, 255, 170, 170, 170, 255, 165, 165, 165, 255, 165, 165, 165, 255, 165, 165, 165, 255, 156, 156, 156, 197, 42, 42, 42, 102, 64, 64, 64, 41, 64, 64, 64, 0, 0, 0, 0, 230, 146, 146, 146, 255, 178, 178, 178, 255, 175, 175, 175, 255, 171, 171, 171, 255, 168, 168, 168, 255, 166, 166, 166, 255, 166, 166, 166, 255, 165, 165, 165, 255, 144, 144, 144, 250, 113, 113, 113, 235, 76, 76, 76, 214, 54, 54, 54, 146, 50, 50, 50, 74, 64, 64, 64, 25, 64, 64, 64, 0, 0, 0, 0, 230, 152, 152, 152, 255, 169, 169, 169, 255, 167, 167, 167, 255, 167, 167, 167, 255, 163, 163, 163, 255, 145, 145, 145, 250, 113, 113, 113, 237, 79, 79, 79, 192, 39, 39, 39, 162, 46, 46, 46, 130, 62, 62, 62, 109, 64, 64, 64, 80, 64, 64, 64, 40, 64, 64, 64, 14, 64, 64, 64, 0, 0, 0, 0, 232, 158, 158, 158, 255, 150, 150, 150, 251, 121, 121, 121, 239, 85, 85, 85, 219, 55, 55, 55, 189, 40, 40, 40, 158, 48, 48, 48, 132, 60, 60, 60, 97, 64, 64, 64, 80, 64, 64, 64, 62, 64, 64, 64, 44, 64, 64, 64, 28, 64, 64, 64, 15, 64, 64, 64, 6, 64, 64, 64, 0, 0, 0, 0, 133, 56, 56, 56, 165, 34, 34, 34, 155, 43, 43, 43, 140, 58, 58, 58, 117, 64, 64, 64, 98, 64, 64, 64, 79, 64, 64, 64, 60, 64, 64, 64, 35, 64, 64, 64, 26, 64, 64, 64, 18, 64, 64, 64, 11, 64, 64, 64, 6, 64, 64, 64, 3, 64, 64, 64, 1, 64, 64, 64, 0, 0, 0, 0, 31, 64, 64, 64, 70, 64, 64, 64, 86, 64, 64, 64, 75, 64, 64, 64, 54, 64, 64, 64, 37, 64, 64, 64, 26, 64, 64, 64, 17, 64, 64, 64, 7, 64, 64, 64, 4, 64, 64, 64, 2, 64, 64, 64, 1, 64, 64, 64, 0, 255, 255, 255, 0, 255, 255, 255, 0, 255, 255, 255, 0, 0, 0, 0], "mask"=[0, 0, 0, 124, 127, 254, 255, 254, 255, 254, 255, 254, 255, 254, 255, 252, 255, 252, 255, 248, 255, 248, 255, 248, 255, 224, 255, 0, 240, 0, 0, 0], "colors"=[], "Rectangle"={"left"=0, "top"=0, "right"=16, "bottom"=16}}, {"image type"=0, "image depth"=32, "image"=[255, 132, 170, 222, 255, 132, 170, 222, 255, 132, 170, 222, 255, 132, 170, 222, 255, 132, 170, 222, 255, 132, 170, 222, 255, 132, 170, 222, 255, 132, 170, 222, 255, 132, 170, 222, 255, 132, 170, 222, 255, 115, 130, 181, 0, 0, 0, 0, 0, 0, 0, 0, 0, 0, 0, 0, 0, 0, 0, 0, 0, 0, 0, 0, 255, 132, 154, 206, 255, 255, 255, 255, 255, 255, 255, 255, 255, 255, 255, 255, 255, 255, 255, 255, 255, 255, 255, 255, 255, 255, 255, 255, 255, 255, 255, 255, 255, 255, 255, 255, 255, 231, 243, 255, 255, 115, 130, 181, 255, 132, 170, 222, 0, 0, 0, 0, 0, 0, 0, 0, 0, 0, 0, 0, 0, 0, 0, 0, 255, 132, 154, 206, 255, 247, 251, 255, 255, 255, 255, 255, 255, 255, 251, 255, 255, 247, 247, 247, 255, 247, 247, 247, 255, 247, 247, 247, 255, 247, 247, 247, 255, 231, 243, 255, 255, 231, 243, 255, 255, 115, 130, 181, 255, 115, 130, 181, 255, 115, 130, 181, 0, 0, 0, 0, 0, 0, 0, 0, 0, 0, 0, 0, 255, 132, 154, 206, 255, 247, 251, 255, 255, 247, 251, 255, 255, 247, 243, 247, 255, 247, 243, 247, 255, 247, 243, 247, 255, 231, 243, 255, 255, 231, 243, 255, 255, 231, 243, 255, 255, 231, 243, 255, 255, 231, 243, 255, 255, 206, 211, 255, 255, 115, 121, 173, 0, 0, 0, 0, 0, 0, 0, 0, 0, 0, 0, 0, 255, 132, 158, 206, 255, 198, 199, 222, 255, 189, 186, 214, 255, 189, 186, 214, 255, 189, 186, 214, 255, 189, 186, 214, 255, 189, 186, 214, 255, 189, 186, 214, 255, 189, 186, 214, 255, 189, 186, 214, 255, 107, 109, 140, 255, 206, 211, 255, 255, 115, 121, 173, 0, 0, 0, 0, 0, 0, 0, 0, 0, 0, 0, 0, 255, 132, 154, 206, 255, 189, 186, 214, 255, 189, 178, 165, 255, 189, 178, 165, 255, 189, 178, 165, 255, 189, 178, 165, 255, 189, 178, 165, 255, 189, 178, 165, 255, 165, 162, 165, 255, 156, 154, 156, 255, 132, 134, 173, 255, 206, 211, 255, 255, 115, 121, 173, 0, 0, 0, 0, 0, 0, 0, 0, 0, 0, 0, 0, 255, 132, 150, 198, 255, 189, 186, 214, 255, 24, 142, 8, 255, 0, 16, 0, 255, 24, 121, 16, 255, 0, 0, 0, 255, 24, 125, 16, 255, 66, 73, 57, 255, 189, 178, 165, 255, 181, 170, 156, 255, 148, 142, 173, 255, 206, 211, 255, 255, 115, 121, 173, 0, 0, 0, 0, 0, 0, 0, 0, 0, 0, 0, 0, 255, 132, 150, 198, 255, 189, 186, 214, 255, 24, 134, 8, 255, 0, 16, 0, 255, 24, 121, 16, 255, 0, 12, 0, 255, 24, 121, 16, 255, 66, 89, 57, 255, 214, 178, 24, 255, 206, 199, 181, 255, 140, 138, 173, 255, 206, 211, 255, 255, 115, 121, 173, 0, 0, 0, 0, 0, 0, 0, 0, 0, 0, 0, 0, 255, 123, 138, 181, 255, 189, 186, 214, 255, 0, 16, 0, 255, 24, 121, 16, 255, 0, 16, 0, 255, 24, 121, 16, 255, 0, 12, 0, 255, 49, 73, 99, 255, 214, 178, 24, 255, 140, 130, 33, 255, 140, 130, 33, 255, 206, 211, 255, 255, 115, 121, 173, 0, 0, 0, 0, 0, 0, 0, 0, 0, 0, 0, 0, 255, 123, 134, 181, 255, 189, 186, 214, 255, 0, 0, 0, 255, 0, 121, 24, 255, 0, 0, 0, 255, 0, 121, 24, 255, 0, 4, 0, 255, 181, 174, 165, 255, 214, 182, 24, 255, 255, 255, 0, 255, 255, 255, 0, 255, 140, 130, 33, 255, 140, 130, 33, 0, 0, 0, 0, 0, 0, 0, 0, 0, 0, 0, 0, 255, 123, 130, 173, 255, 189, 186, 214, 255, 181, 178, 165, 255, 181, 178, 165, 255, 181, 178, 165, 255, 181, 178, 165, 255, 255, 0, 0, 255, 255, 0, 0, 255, 214, 182, 24, 255, 255, 255, 0, 255, 107, 101, 33, 255, 255, 255, 0, 255, 255, 255, 0, 255, 140, 130, 33, 0, 0, 0, 0, 0, 0, 0, 0, 255, 123, 125, 173, 255, 189, 186, 214, 255, 181, 178, 165, 255, 181, 178, 165, 255, 181, 178, 165, 255, 181, 178, 165, 255, 181, 178, 165, 255, 181, 178, 165, 255, 214, 182, 24, 255, 107, 101, 33, 255, 0, 0, 0, 255, 107, 101, 33, 255, 255, 255, 0, 255, 255, 0, 0, 255, 255, 0, 0, 0, 0, 0, 0, 255, 115, 121, 165, 255, 181, 182, 214, 255, 123, 121, 140, 255, 123, 121, 140, 255, 123, 121, 140, 255, 123, 121, 140, 255, 0, 0, 255, 255, 0, 0, 255, 255, 214, 182, 24, 255, 255, 255, 0, 255, 107, 101, 33, 255, 255, 255, 0, 255, 255, 255, 0, 255, 99, 93, 49, 0, 0, 0, 0, 0, 0, 0, 0, 255, 115, 121, 165, 255, 206, 211, 255, 255, 206, 211, 255, 255, 206, 211, 255, 255, 206, 211, 255, 255, 206, 211, 255, 255, 206, 211, 255, 255, 206, 211, 255, 255, 214, 182, 24, 255, 255, 255, 0, 255, 255, 255, 0, 255, 140, 130, 33, 255, 140, 130, 33, 0, 0, 0, 0, 0, 0, 0, 0, 0, 0, 0, 0, 255, 115, 121, 173, 255, 115, 121, 173, 255, 115, 121, 173, 255, 115, 121, 173, 255, 115, 121, 173, 255, 115, 121, 173, 255, 115, 121, 173, 255, 115, 121, 173, 255, 206, 182, 66, 255, 148, 134, 33, 255, 140, 130, 33, 255, 115, 121, 173, 255, 115, 121, 173, 0, 0, 0, 0, 0, 0, 0, 0, 0, 0, 0, 0, 0, 0, 0, 0, 0, 0, 0, 0, 0, 0, 0, 0, 0, 0, 0, 0, 0, 0, 0, 0, 0, 0, 0, 0, 0, 0, 0, 0, 0, 0, 0, 0, 0, 0, 0, 0, 0, 0, 0, 0, 0, 0, 0, 0, 0, 0, 0, 0, 0, 0, 0, 0, 0, 0, 0, 0, 0, 0, 0, 0, 0, 0, 0, 0], "mask"=[255, 224, 255, 240, 255, 248, 255, 248, 255, 248, 255, 248, 255, 248, 255, 248, 255, 248, 255, 248, 255, 252, 255, 254, 255, 252, 255, 248, 255, 248, 0, 0], "colors"=[], "Rectangle"={"left"=0, "top"=0, "right"=16, "bottom"=16}}] ("Array")) -> (error out=w66:errorcluster)  [unwired: 3 in, 3 out]
        n15 = property on="_IconSize" class="Ring (strict)"("Value"=w64, "Visible"=FALSE) -> ()  [unwired: 2 in, 2 out]
        n16 = invoke on="Tree" class="Tree (strict)" method="Edit Tree Items.Delete"(error in=w66) -> ()  [unwired: 4 in, 5 out]
        n17 = control-ref of="FloodFillMask"() -> (w57:refnum<vi>)
        n18 = control-ref of="_IconSearchText"() -> (w56:refnum<vi>)
        n19 = control-ref of="_Manage"() -> (w55:refnum<vi>)
        n20 = control-ref of="_Folders"() -> (w54:refnum<vi>)
        n21 = control-ref of="Icons"() -> (w53:refnum<vi>)
        n22 = property on="Ballon" class="Clust (strict)"("Visible"=FALSE) -> ()  [unwired: 2 in, 2 out]
        n23 = Build Array(w57, w56, w55, w54, w53) -> (w52:refnum<vi>[])
        n24 = for {
          tunnel: w52 -> [w75] mode=indexing
          n25 = property class="Ctl"(reference=w75, "Visible"=FALSE) -> ()  [unwired: 1 in, 2 out]
        }
        n26 = local write "_IconSearchText"("" ("_IconSearchText")) -> ()
        n27 = local write "_HideHeader"(FALSE ("_HideHeader")) -> ()
        n28 = local write "_TextAlignment"(w62) -> ()
        n29 = local write "_BodyBk"(T2 {"Decal"=FALSE, "Color"=16774466} ("_BodyBk")) -> ()
        n30 = local write "_BodyText"(T2 {"Decal"=FALSE, "Color"=0} ("_BodyText")) -> ()
        n31 = local write "_FontCompression"(enum16{"Auto", "On", "Off"}."Auto" ("_FontCompression")) -> ()
        n32 = local write "_CapitalOnly"(TRUE ("_CapitalOnly")) -> ()
        n33 = property on="_MethodIcons" class="Bool"("Visible"=TRUE) -> ()  [unwired: 2 in, 2 out]
        n34 = First Call?() -> (First Call?: T/F=w46:bool)
        n35 = case shown="True" w46 {
          frame False {
          }
          frame True {
            n36 = local write "FloodFillMask"(TRUE ("_CapitalOnly")) -> ()
          }
        }
        n37 = Tick Count (ms)() -> (millisecond timer value=w47:u32)
        n38 = Bundle By Name(cluster=w68, "StartTime"=w47, "ClassIndex"=0 ("Counter")) -> (w70:T5)
        "Ballon" <- cluster{"format string":string} {"format string"="There are more VIs with the same name found in sibling classes.\nBy default all of them will be renamed.\nYou can double click on VIs to control if they should or shouldn't be renamed."} ("Ballon")
      }
      frame "GetViInfo" {
        w95 = T2 {"Decal"=FALSE, "Color"=56339} ("_BodyBk")
        w105 = u8 32 ("x")
        n39 = property class="ProjectItem"(reference=w133, error in=w102) -> (error out=w84:errorcluster, "Path"=w118:path, "Reference"=w87:refnum<vi>)  [unwired: 1 out]
        "_VIPath" <- w118
        n40 = Unbundle By Name(w134) -> ()  [unwired: 1 out]
        n41 = property class="VI"(reference=w87, error in=w84) -> (reference out=w126:refnum<vi>, error out=w103:errorcluster, "Library"=w129:refnum<vi>)
        n42 = invoke class="VI" method="VI Icon.Get as Image Data"(reference=w87, error in=w84) -> (reference out=w86:refnum<vi>, error out=w83:errorcluster, "ImageData"=w88:T4)  [unwired: 4 in, 3 out]
        n43 = property class="Library"(reference=w129, error in=w103) -> (reference out=w125:refnum<vi>, "Type String"=w128:string, "Path"=w122:path)  [unwired: 1 out]
        n44 = call <vilib>:"Draw Flattened Pixmap.vi"("image data"=w88) -> ("new picture"=→"_Before":picture)  [unwired: 8 in]
        n45 = call <resource>:"GDSLvIcon_AnalyseViIcon.vi"("ViRef/LvCLassRef/LvLibRef/ViPath/2D_Image"=w86, "error in (no error)"=w83) -> ("BodyTextColor"=w78:u32, "FrameColor"=w97:u32, "FrameThickness(1)"=w98:u32, "ValidHeaderIcon"=w91:bool, "DefaultIcon"=w79:bool, "HeaderIcon"=w99:u8[][], "HeaderBkColor"=w101:u32, "BodyIcon"=w81:u8[][], "BodyBkColor"=w100:u32, "error out"=w104:errorcluster)  [unwired: 5 in, 3 out]
        n46 = Not A Number/Path/Refnum?(number/path/refnum=w125) -> (NaN/Path/Refnum?=w132:bool)
        n47 = Not Equal?(x=w128, y="LVClass") -> (x != y?=w123:bool)
        n48 = And(x=w132, y=w123) -> (x .and. y?=w124:bool)
        n49 = Strip Path(path=w118) -> (name=w77:string)  [unwired: 1 out]
        n50 = call <vilib>:"Get File Extension.vi"("file"=w118) -> ("filename without extension"=w89:string, "lowercase file extension"=w76:string)  [unwired: 6 in, 3 out]
        n51 = case shown="True" w79 {
          tunnel: [w140 u32 0] -> w117
          tunnel: [w139 w152] -> w116
          tunnel: w100 -> [w137 _]
          tunnel: w78 -> [w136 _]
          tunnel: w81 -> [w135 _]
          tunnel: w80 -> [_ w151]
          frame False {
            n52 = Equal?(x=w137, y=w136) -> (x = y?=w138:bool)
            n53 = Equal?(x=w136, y=u32 0) -> (x = y?=w141:bool)
            n54 = case shown="False" w138 {
              tunnel: w136 -> [w143 _]
              tunnel: w137 -> [w144 w149]
              tunnel: [w144 w149] -> w139
              tunnel: [w143 w147] -> w140
              tunnel: w141 -> [_ w148]
              tunnel: w135 -> [_ _]
              frame False {
              }
              frame True {
                n55 = Select(t=u32 16777215, s=w148, f=u32 0) -> (s? t:f=w147:u32)
              }
            }
          }
          frame True {
            n56 = Random Number (0-1)() -> (number: 0 to 1=w154:dbl)
            n57 = Array Size(array=w151) -> (size(s)=w150:i32)
            n58 = Multiply(x=w150, y=w154) -> (x*y=w155:dbl)
            n59 = Round Toward -Infinity(1:w155) -> (0:w153:dbl)
            n60 = Index Array(array=w151, index=w153) -> (element=w152:u32)
          }
        }
        n61 = String Length(string=w89) -> (length=w119:i32)
        n62 = Array Size(array=w99) -> (size(s)=w106:i32[])
        n63 = property on="NewName" class="Str"("Value"=w89, "Key Focus"=TRUE, "Text.Selection Start"=u32 0 ("Text.Selection:Start"), "Text.Selection End"=w119) -> ()  [unwired: 2 in, 2 out]
        n64 = Index Array(array=w106) -> (element #1=w111:i32)  [unwired: 2 in, 1 out]
        n65 = Multiply(x=w98, y=u8 2) -> (x*y=w110:u32)
        n66 = Equal To 0?(x=w111) -> (x = 0?=w112:bool)
        n67 = Add(x=w111, y=w110) -> (x+y=w114:u32)
        n68 = Bundle(cluster=w95, "Color"=w116) -> (w96:T2)  [unwired: 1 in]
        n69 = Bundle(cluster=w95, "Color"=w117) -> (w94:T2)  [unwired: 1 in]
        n70 = Increment(x=w114) -> (x+1=w113:u32)
        n71 = Select(t=w114, s=w112, f=w113) -> (s? t:f=w115:u32)
        n72 = local write "_MethodIconName"(w89) -> ()
        n73 = Bundle By Name(cluster=w134, "VIPath"=w118, "VIref"=w126, "Class"=w125, "ClassPath"=w122, "NewName"=w77, "FileExtension"=w76) -> (w93:T5)
        n74 = local write "_BodyText"(w94) -> ()
        n75 = Subtract(x=w105, y=w115) -> (x-y=w107:u32)
        n76 = Subtract(x=w105, y=w110) -> (x-y=w108:u32)
        n77 = local write "_BodyBk"(w96) -> ()
        n78 = Bundle By Name(cluster=w93, "FrameColor"=w97, "Frame thickness"=w98, "HeaderIcon"=w99, "BodyIconHeight"=w107, "BodyIconWidth"=w108, "Header exists"=w91, "HeaderBkColor"=w101) -> (w92:T5)
        n79 = property on="_HideHeader" class="Bool (strict)"("Visible"=w91, "Value"=FALSE ("_HideHeader")) -> ()  [unwired: 2 in, 2 out]
        n80 = Select(t="UpdateIcons", s=w124, f="GoThoughClassHierarchy") -> (s? t:f=w130:string)
      }
      frame "GoThoughClassHierarchy" {
        w160 = refnum<vi> refnum  # LVClassLibrary
        w177 = refnum<vi> refnum  # LVClassLibrary
        w182 = TRUE ("ExcludeDependencies")
        n81 = Unbundle By Name(w165) -> ("Class"=w176:refnum<vi>)
        n82 = To More Specific Class(target class=w177, reference=w176) -> (specific class reference=w175:refnum<vi>)  [unwired: 1 in, 1 out]
        n83 = Unbundle By Name(w165) -> ()  [unwired: 1 out]
        n84 = call <resource>:"GDSLvClass_GetRootBaseClass.vi"("ViRef/Path,LvClassRef/Path"=w175, "error in (no error)"=w159, "LimitToSpecificProviderTypeOfSameType(True)"=FALSE) -> ("RootBaseClassPath"=w164:path, "error out"=w170:errorcluster)  [unwired: 11 in, 4 out]
        n85 = property class="ProjectItem"(reference=w166, error in=w170) -> (error out=w171:errorcluster, "Target"=w173:refnum<vi>, "Project"=w169:refnum<vi>)  [unwired: 1 out]
        n86 = Not A Number/Path/Refnum?(number/path/refnum=w173) -> (NaN/Path/Refnum?=w167:bool)
        n87 = case shown="False" w167 {
          tunnel: w169 -> [w185 w192]
          tunnel: [w187 w189] -> w174
          tunnel: w173 -> [w187 _]
          tunnel: [w186 w191] -> w172
          tunnel: w159 -> [_ w190]
          tunnel: w171 -> [w186 _]
          tunnel: [w185 w188] -> w161
          frame False {
          }
          frame True {
            n88 = property class="Project"(reference=w192, error in=w190) -> (reference out=w188:refnum<vi>, error out=w191:errorcluster, "My Computer"=w189:refnum<vi>)
          }
        }
        n89 = invoke class="TargetItem" method="Get All Descendents"(reference=w174, error in=w172, "Type"="LvClass", "Exclude Dependencies"=w182, "ExcludeBuilds"=w182, "ExcludeTargets"=w182) -> (reference out=w180:refnum<vi>, error out=w181:errorcluster, "All Descendents"=w178:refnum<vi>[])  [unwired: 1 in, 4 out]
        n90 = Close Reference(reference=w180, error in (no error)=w181) -> (error out=w179:errorcluster)
        n91 = Close Reference(reference=w161) -> ()  [unwired: 1 in, 1 out]
        n92 = for {
          tunnel: w178 -> [w197] mode=indexing
          tunnel: [w205] -> w163 mode=indexing if=w201
          tunnel: w164 -> [w203]
          tunnel: w160 -> [w195]
          shift-right: [w193] -> w158
          shift-left: w179 -> [w198]
          n93 = To More Specific Class(target class=w195, reference=w197, error in=w198) -> (specific class reference=w196:refnum<vi>, error out=w194:errorcluster)
          n94 = while {
            shift-right: [w214] -> _
            shift-left: w196 -> [w207]
            shift-right: [w213] -> w193
            shift-left: w194 -> [w206]
            tunnel: [w212] -> w200 mode=indexing
            tunnel: [w210] -> w204 mode=indexing
            i -> [w209]
            stop <- w211 stop-if-true
            n95 = property class="LVClassLibrary"(reference=w207, error in=w206) -> (reference out=w216:refnum<vi>, error out=w215:errorcluster, "Path"=w210:path, "Name"=w218:string, "QualifiedName"=w217:string)
            n96 = Bundle("Path"=w210, "Name"=w218, "QualifiedName"=w217) -> (w212:T15)  [unwired: 1 in]
            n97 = property class="LVClassLibrary"(reference=w216, error in=w215) -> (reference out=w208:refnum<vi>, error out=w213:errorcluster, "Parent"=w214:refnum<vi>)
            n98 = case shown="1.." w209 {
              tunnel: w208 -> [_ w219]
              frame 0, Default {
              }
              frame 1.. {
                n99 = Close Reference(reference=w219) -> ()  [unwired: 1 in, 1 out]
              }
            }
            n100 = Not A Number/Path/Refnum?(number/path/refnum=w214) -> (NaN/Path/Refnum?=w211:bool)
          }
          n101 = Search 1D Array(1D array=w204, element=w203) -> (index of element=w202:i32)  [unwired: 1 in]
          n102 = Greater Or Equal To 0?(x=w202) -> (x >= 0?=w201:bool)
          n103 = Array Size(array=w200) -> (size(s)=w199:i32)
          n104 = Bundle(w199, w196, w200) -> (w205:T16)  [unwired: 1 in]
        }
        n105 = Sort 1D Array(array=w163) -> (sorted array=w157:T17)
        n106 = Bundle By Name(cluster=w165, "Classes"=w157) -> (w162:T5)
      }
      frame "FindViInClasses" {
        n107 = Unbundle By Name(w223) -> ("Classes"=w233:T17, "VIPath"=w232:path)
        n108 = Strip Path(path=w232) -> (name=w231:string)  [unwired: 1 out]
        n109 = To Lower Case(string=w231) -> (all lower case string=w230:string)
        n110 = for {
          tunnel: w233 -> [w257] mode=indexing
          tunnel: w230 -> [w253]
          shift-right: [w244] -> w228
          shift-left: w229 -> [w247]
          tunnel: [w240] -> w226 mode=indexing
          tunnel: [w237] -> w224 mode=indexing
          w256 = TRUE ("ExcludeDependencies")
          n111 = Unbundle(w257) -> (w254:refnum<vi>, w252:T18)  [unwired: 1 out]
          n112 = Index Array(array=w252) -> (element=w251:T15)  [unwired: 1 in]
          n113 = Unbundle By Name(w251) -> ("Path"=w249:path)
          n114 = invoke class="LVClassLibrary" method="Get All Descendents"(reference=w254, error in=w247, "Type"="VI", "Exclude Dependencies"=w256, "ExcludeBuilds"=w256, "ExcludeTargets"=w256) -> (reference out=w235:refnum<vi>, error out=w248:errorcluster, "All Descendents"=w245:refnum<vi>[])  [unwired: 1 in, 4 out]
          n115 = Strip Path(path=w249) -> (stripped path=w250:path)  [unwired: 1 out]
          n116 = call <vilib>:"Get File Extension.vi"("file"=w249) -> ("filename without extension"=w237:string)  [unwired: 6 in, 4 out]
          n117 = for {
            tunnel: w245 -> [w275] mode=indexing
            tunnel: w253 -> [w273]
            tunnel: [w272] -> w239 if=w261
            shift-right: [w267] -> w246
            shift-left: w248 -> [w271]
            tunnel: [w265] -> w242 mode=indexing
            tunnel: [w270] -> w236 if=w261
            tunnel: w235 -> [w268]
            tunnel: [w262] -> w234 if=w261
            n118 = property class="ProjectItem"(reference=w275, error in=w271) -> (reference out=w266:refnum<vi>, error out=w269:errorcluster, "Path"=w270:path)
            n119 = Strip Path(path=w270) -> (stripped path=w272:path, name=w265:string)
            n120 = To Lower Case(string=w265) -> (all lower case string=w274:string)
            n121 = invoke class="LVClassLibrary" method="Get Source Scope"(reference=w268, error in=w269, "SourceRef"=w266) -> (error out=w267:errorcluster, "GetSourceScope"=w264:T8)  [unwired: 2 in, 3 out]
            n122 = Equal?(x=w274, y=w273) -> (x = y?=w261:bool)
            n123 = Equal?(x=T8."private" ("y"), y=w264) -> (x = y?=w262:bool)
          }
          n124 = Empty String/Path?(string/path=w239) -> (empty?=w238:bool)
          n125 = case shown="False" w238 {
            tunnel: w250 -> [w260 _]
            tunnel: [w259 _] -> w243
            tunnel: w239 -> [w258 _]
            frame False {
              n126 = call <vilib>:"Compare Two Paths.vi"("Path 2"=w258, "Path 1"=w260) -> ("Relative Path from 1 to 2"=w259:path)  [unwired: 6 in, 3 out]
            }
            frame True {
            }
          }
          n127 = Close Reference(reference=w245, error in (no error)=w246) -> (error out=w244:errorcluster)
          n128 = Bundle(cluster=T7 {"ClassName"="", "ViRelPath"=path "", "AllVIs"=[], "VI-Path"=path "", "Private"=FALSE}, "ClassName"=w237, "ViRelPath"=w243, "AllVIs"=w242, "VI-Path"=w236, "Private"=w234) -> (w240:T7)
        }
        n129 = Unbundle By Name(w223) -> ("ClassPath"=w222:path)
        n130 = call <vilib>:"Get File Extension.vi"("file"=w222) -> ("filename without extension"=w221:string)  [unwired: 6 in, 4 out]
        n131 = Search 1D Array(1D array=w224, element=w221) -> (index of element=w220:i32)  [unwired: 1 in]
        n132 = Bundle By Name(cluster=w223, "ClassIndex"=w220, "ClassInfos"=w226) -> (w227:T5)
      }
      frame "CreateClassList" {
        n133 = Unbundle By Name(w289) -> ("ClassIndex"=w276:i32, "ClassInfos"=w288:T19, "VIPath"=w287:path)
        n134 = Strip Path(path=w287) -> (name=w286:string)  [unwired: 1 out]
        n135 = for {
          tunnel: w288 -> [w314] mode=indexing
          shift-right: [w302] -> w284
          shift-left: w285 -> [w310]
          tunnel: w286 -> [w304]
          tunnel: [w299] -> w280 mode=indexing
          tunnel: [w294] -> w281 mode=indexing if=w297
          tunnel: w276 -> [w293]
          i -> [w294]
          n136 = Unbundle By Name(w314) -> ("Private"=w291:bool, "ViRelPath"=w301:path, "ClassName"=w298:string)
          n137 = Not Equal?(x=w294, y=w293) -> (x != y?=w292:bool)
          n138 = invoke on="Tree" class="Tree (strict)" method="Edit Tree Items.Add Item"(error in=w310, "Child Position"=-1, "Left Cell"=w298, "Child Tag"=w298) -> (error out=w311:errorcluster, "Edit Tree Items:Add Item"=w309:string)  [unwired: 5 in, 7 out]
          n139 = Path To String(path=w301) -> (string=w300:string)
          n140 = And(x=w292, y=w291) -> (x .and. y?=w290:bool)
          n141 = property on="Tree" class="Tree (strict)"(error in=w311, "Active Item Tag"=w309, "Glyph"=1 ("Active Item:Symbol Index")) -> (error out=w308:errorcluster)  [unwired: 1 in, 1 out]
          n142 = Format Into String(format string="%s:VI", w298) -> (resulting string=w303:string)  [unwired: 2 in, 1 out]
          n143 = case shown="\"\", \".\"" w300 {
            selector: w300 -> [w328 _]
            tunnel: w309 -> [w329 w333]
            tunnel: w308 -> [w327 w332]
            tunnel: [w326 w333] -> w306
            tunnel: [w325 w332] -> w307
            frame Default {
              n144 = invoke on="Tree" class="Tree (strict)" method="Edit Tree Items.Add Item"(error in=w327, "Parent Tag"=w329, "Left Cell"=w328) -> (error out=w331:errorcluster, "Edit Tree Items:Add Item"=w326:string)  [unwired: 6 in, 7 out]
              n145 = property on="Tree" class="Tree (strict)"(error in=w331, "Active Item Tag"=w326, "Glyph"=2 ("Active Item:Symbol Index")) -> (error out=w325:errorcluster)  [unwired: 1 in, 1 out]
            }
            frame "", "." {
            }
          }
          n146 = Empty String/Path?(string/path=w300) -> (empty?=w296:bool)
          n147 = case shown="False" w296 {
            tunnel: w307 -> [w319 w324]
            tunnel: w306 -> [w318 _]
            tunnel: w304 -> [w317 _]
            tunnel: w303 -> [w315 _]
            tunnel: [w316 w324] -> w302
            tunnel: [w315 ""] -> w299
            tunnel: w298 -> [_ _]
            frame False {
              n148 = invoke on="Tree" class="Tree (strict)" method="Edit Tree Items.Add Item"(error in=w319, "Parent Tag"=w318, "Left Cell"=w317, "Child Tag"=w315) -> (error out=w320:errorcluster, "Edit Tree Items:Add Item"=w322:string)  [unwired: 5 in, 7 out]
              n149 = property on="Tree" class="Tree (strict)"(error in=w320, "Active Item Tag"=w322, "Glyph"=3 ("Active Item:Symbol Index")) -> (error out=w316:errorcluster)  [unwired: 1 in, 1 out]
            }
            frame True {
            }
          }
          n150 = Or(x=w290, y=w296) -> (x .or. y?=w295:bool)
          n151 = Not(x=w295) -> (.not. x?=w297:bool)
        }
        n152 = Bundle By Name(cluster=w289, "Selected"=w281, "TreeTags"=w280) -> (w282:T5)
        n153 = Array Size(array=w280) -> (size(s)=w279:i32)
        n154 = Greater?(x=w279, y=1) -> (0:w277:bool)
        n155 = property on="Ballon" class="Clust (strict)"("Visible"=w277) -> ()  [unwired: 2 in, 2 out]
      }
      frame "UpdateClassList" {
        (unwired) u32 12303291
        n156 = Unbundle By Name(w348) -> ("VIPath"=w343:path, "Classes"=w347:T17, "ClassInfos"=w346:T19, "TreeTags"=w345:string[], "NewName"=w344:string, "ClassIndex"=w339:i32, "Selected"=w342:i32[])
        n157 = Strip Path(path=w343) -> (name=w341:string)  [unwired: 1 out]
        n158 = for {
          tunnel: w347 -> [_] mode=indexing
          tunnel: w346 -> [w357] mode=indexing
          tunnel: w345 -> [w351] mode=indexing
          tunnel: w344 -> [w363]
          tunnel: w342 -> [w362]
          tunnel: w341 -> [w358]
          tunnel: w339 -> [w353]
          tunnel: [w350] -> w338 mode=indexing
          i -> [w354]
          n159 = Equal?(x=w354, y=w353) -> (x = y?=w352:bool)
          n160 = Search 1D Array(1D array=w362, element=w354) -> (index of element=w359:i32)  [unwired: 1 in]
          n161 = Unbundle(w357) -> ("AllVIs"=w356:string[])  [unwired: 4 out]
          n162 = To Lower Case(string=w356) -> (all lower case string=w355:string[])
          n163 = case shown="-1" w359 {
            tunnel: w363 -> [w376 _]
            tunnel: [w374 w399] -> w361
            tunnel: [w373 u32 16777216] -> w360
            tunnel: w358 -> [_ w399]
            tunnel: w355 -> [w372 _]
            tunnel: w352 -> [w371 _]
            tunnel: [w370 _] -> w350
            frame 0, Default {
              n164 = Empty String/Path?(string/path=w376) -> (empty?=w375:bool)
              n165 = case shown="True" w375 {
                tunnel: w376 -> [_ w382]
                tunnel: ["(Can't be empty)" w387] -> w374
                tunnel: [u32 16711680 w386] -> w373
                tunnel: w372 -> [_ w384]
                tunnel: w371 -> [_ w381]
                tunnel: [TRUE w380] -> w370
                frame True {
                }
                frame False {
                  n166 = To Lower Case(string=w382) -> (all lower case string=w385:string)
                  n167 = Search 1D Array(1D array=w384, element=w385) -> (index of element=w383:i32)  [unwired: 1 in]
                  n168 = case shown="-1" w383 {
                    tunnel: [w392 w394] -> w387
                    tunnel: [w389 u32 16711680] -> w386
                    tunnel: w382 -> [w392 w396]
                    tunnel: w381 -> [w391 _]
                    tunnel: [_ TRUE] -> w380
                    frame -1 {
                      n169 = Select(t=u32 12303291, s=w391, f=u32 12124108) -> (s? t:f=w389:u32)
                    }
                    frame Default {
                      n170 = Format Into String(format string="%s (Exists)", w396) -> (resulting string=w394:string)  [unwired: 2 in, 1 out]
                    }
                  }
                }
              }
            }
            frame -1 {
            }
          }
          n171 = case shown="Default" w351 {
            selector: w351 -> [_ w364]
            tunnel: w361 -> [_ w366]
            tunnel: w360 -> [_ w365]
            frame "" {
            }
            frame Default {
              n172 = property on="Tree" class="Tree (strict)"("Active Item Tag"=w364) -> (error out=w368:errorcluster)  [unwired: 2 in, 1 out]
              n173 = property on="Tree" class="Tree (strict)"(error in=w368, "Cell String"=w366) -> (error out=w367:errorcluster)  [unwired: 1 in, 1 out]
              n174 = property on="Tree" class="Tree (strict)"(error in=w367, "ActiveColNum"=0 ("Active Cell:Active Column Number"), "CellBG"=w365) -> ()  [unwired: 1 in, 2 out]
            }
          }
        }
        n175 = Or Array Elements(Boolean array=w338) -> (logical OR=w337:bool)
        n176 = Select(t=T9."Disabled and Grayed Out" ("Disabled"), s=w337, f=T9."Enabled" ("Disabled")) -> (s? t:f=w334:T9)
        n177 = property on="_RenameVI" class="Bool"("DisabledEnum"=w334) -> ()  [unwired: 2 in, 2 out]
      }
      frame "Generate icon", "UpdateIcons" {
        n178 = Unbundle By Name(w401) -> ("CurrentIcon"=w445:T20)
        n179 = Unbundle By Name(w401) -> ("ConnectorPaneHeight"=w441:i32[], "BodyIconHeight"=w442:i32, "BodyIconWidth"=w444:i32)
        n180 = Unbundle By Name(w401) -> ("StartIconSize"=w423:u16, "StartRow"=w426:i32, "FrameColor"=w419:u32, "Frame thickness"=w420:i32, "HeaderIcon"=w421:u8[][])
        n181 = local read "_IconSize"() -> (w408:u16)
        n182 = local read "_HideHeader"() -> (w443:bool)
        n183 = local read "_BodyBk"() -> (w406:T2)
        n184 = Unbundle By Name(w401) -> ("HeaderBkColor"=w400:u32)
        n185 = Unbundle By Name(w406) -> ("Color"=w402:u32)
        n186 = call <resource>:"GDSIconEditor_IconSizeAdjustment.vi"("BodyIconHeightIn"=w442, "HideHeader"=w443, "ConnectorPaneHeight"=w441, "Frame thickness"=w420, "_IconSize"=w408, "HeaderIconIn"=w421) -> ("HeaderIconOut"=w440:u8[][], "BodyIconHeightOut"=w439:u32, "ImageRows"=w438:i32)  [unwired: 3 in]
        n187 = Not Equal?(x=w423, y=w408) -> (x != y?=w424:bool)
        n188 = call <resource>:"GDSLvIcon_Convert24bitTo8bitColor.vi"("Color 24bit In"=w400) -> ("Color out(256)"=w407:u8)  [unwired: 15 in, 3 out]
        n189 = call <resource>:"GDSLvIcon_Convert24bitTo8bitColor.vi"("Color 24bit In"=w402) -> ("Color out(256)"=w405:u8)  [unwired: 15 in, 3 out]
        n190 = Select(t=0, s=w424, f=w426) -> (s? t:f=w409:i32)
        n191 = local read "_FontCompression"() -> (w450:enum16{"Auto", "On", "Off"})
        n192 = local read "_MethodIconName"() -> (w433:string)
        n193 = local read "_CapitalOnly"() -> (w449:bool)
        n194 = local read "_TextAlignment"() -> (w448:u16)
        n195 = Build Array(w407, w405) -> (w403:u8[])
        n196 = local read "_BodyText"() -> (w446:T2)
        n197 = Unbundle By Name(w401) -> ("OldOffset.X"=w428:i32, "OldOffset.Y"=w431:i32)  [unwired: 1 out]
        n198 = Unbundle By Name(w401) -> ("Offset"=w412:cluster{"X":i32, "Y":i32})
        n199 = Bundle By Name(cluster=w445, "ColorsOkayforiconToBeOnTopOf"=w403) -> (w404:T20)
        n200 = Bundle By Name(cluster=T10 {"Text"="", "Allow Only Capital Chars"=FALSE, "Compression"=enum."Auto", "Alignment"=enum."Center"} ("Text"), "Alignment"=w448, "Text"=w433, "Allow Only Capital Chars"=w449, "Compression"=w450) -> (w434:T10)
        n201 = Unbundle(w446) -> ("Color"=w455:u32)  [unwired: 1 out]
        n202 = Unbundle By Name(w412) -> ("X"=w429:i32, "Y"=w432:i32)
        n203 = call <resource>:"GDSLvIcon_GenerateIconText.vi"("Text"=w434, "TextPixelHeight(5-30)"=w439, "Foreground color"=w455, "Background color"=w402, "error in (no error)"=w447, "Offset"=w412, "Text Pixel width(32-FrameThicknes*2))"=w444) -> ("X-Limited"=w417:bool, "Y-Limited"=w416:bool, "TextOut"=w413:u8[][], "TextBounds"=w435:T21, "error out"=w457:errorcluster)  [unwired: 8 in]
        n204 = Select(t=w428, s=w417, f=w429) -> (s? t:f=w427:i32)
        n205 = Select(t=w431, s=w416, f=w432) -> (s? t:f=w430:i32)
        n206 = call <resource>:"GDSLvIcon_CreateIconPicture.vi"("FrameColor"=w419, "FrameThickness(1)"=w420, "HeaderIconIn"=w440, "BodyIconIn"=w413, "error in (no error)"=w457, "ImageRows(32)"=w438, "BigSizeIcon(x6)"=4, "RowStart(0)"=w409, "BgIcon"=w404) -> ("IconPictureOut"=→"_After":picture, "LargeIconPictureOut(x6)"=→"_IconPreview":picture, "BodyOffset"=w451:cluster{"X":i32, "Y":i32}, "error out"=w411:errorcluster)  [unwired: 5 in, 2 out]
        n207 = Unbundle(w451) -> ("X"=w452:i32, "Y"=w453:i32)
        n208 = Bundle("Y"=w453, "X"=w452, "Y"=w453, "X"=w452) -> (w454:cluster{"Y":i32, "X":i32, "Y":i32, "X":i32})  [unwired: 1 in]
        n209 = Add(x=w454, y=w435) -> (x+y=w414:cluster{i32, i32, i32, i32})
        n210 = Bundle By Name(cluster=w401, "Offset.X"=w427, "Offset.Y"=w430, "Icon exist"=TRUE, "BodyIcon"=w413, "TextBounds"=w414) -> (w418:T5)
      }
      frame "", "Idle" {
        n211 = event shown="[20] \"Help\": Value Change" {
          selector: _ -> [_ _ _ _ _ _ _ _ _ _ _ _ _ _ _ _ _ _ _ _ _ _]
          dyn-events: _ -> [_ _ _ _ _ _ _ _ _ _ _ _ _ _ _ _ _ _ _ _ _ _]
          timeout: _ -> [_ _ _ _ _ _ _ _ _ _ _ _ _ _ _ _ _ _ _ _ _ _]
          tunnel: w458 -> [w469 w479 w493 w507 w515 w520 w524 w562 w616 w622 w624 w628 w682 w687 w697 w699 w748 w752 w787 w793 w796 w797]
          tunnel: [w468 w477 w493 w505 w513 w520 w523 w561 w616 w622 w624 w627 w681 w686 w696 w698 w748 w753 w786 w792 w796 w797] -> w461
          tunnel: ["UpdateClassList" "GetImageData" ("y") "UpdateIconFolderList" "Exit" "UpdateIcon,Exit" "DrawIcons:NoBusy" ("y") w522 w563 "ReadIcons" w618 "UpdateIcons" w626 _ _ _ w702 _ w754 "Exit" "UpdateIcon" ("y") _ _] -> w460
          tunnel: w458 -> [w463 _ _ _ w512 _ w526 w560 _ _ _ w625 w683 w688 _ w701 w747 w751 _ w790 _ _]
          event "NewName": Value Change {
            n212 = event-data() -> ()  [unwired: 1 in, 1 out]
            n213 = Unbundle By Name(w463) -> ("FileExtension"=w462:string)
            n214 = call <vilib>:"Trim Whitespace.vi"("string"="NewName") -> ("trimmed string"=w465:string)  [unwired: 1 in]
            n215 = Empty String/Path?(string/path=w465) -> (empty?=w464:bool)
            n216 = case shown="False" w464 {
              tunnel: [w474 _] -> w466
              tunnel: w465 -> [w473 _]
              tunnel: w462 -> [w471 _]
              frame False {
                n217 = Match Pattern(string=w473, regular expression="\\2E[A-Za-z]+$") -> (before substring=w472:string)  [unwired: 1 in, 3 out]
                n218 = local write "_MethodIconName"(w472) -> ()
                n219 = Concatenate Strings(w472, "." ("string"), w471) -> (w474:string)
              }
              frame True {
              }
            }
            n220 = Bundle By Name(cluster=w469, "NewName"=w466) -> (w468:T5)
          }
          event "DragIcon": Mouse Down {
            n221 = event-data() -> ("Coords"=w480:T3)  [unwired: 1 in]
            n222 = property on="DragIcon" class="Pict"() -> ("Draw Area Size"=w482:T22)  [unwired: 2 in, 2 out]
            n223 = Divide(x=w482, y=2) -> (x/y=w484:cluster{"Width":dbl, "Height":dbl})
            n224 = property on="_IconPreview" class="Pict"() -> ("Position"=w486:T13)  [unwired: 2 in, 2 out]
            n225 = Subtract(x=w480, y=w484) -> (x-y=w490:cluster{dbl, dbl})
            n226 = Add(x=w486, y=T13 {"Left"=0, "Top"=16}) -> (x+y=w487:T13)
            n227 = Subtract(x=w490, y=w487) -> (x-y=w489:cluster{dbl, dbl})
            n228 = Divide(x=w489, y=u8 4 ("Disabled")) -> (x/y=w491:cluster{dbl, dbl})
            n229 = property on="DragIcon" class="Pict"("Position"=w490, "Visible"=TRUE) -> ()  [unwired: 2 in, 2 out]
            n230 = Bundle By Name(cluster=w479, "DraggingIcon"=TRUE ("Draging"), "BgIconOffset"=w491) -> (w477:T5)
          }
          event "_MethodIcons": Value Change {
            n231 = event-data() -> ()  [unwired: 1 in, 1 out]
            n232 = control-ref of="FloodFillMask"() -> (w501:refnum<vi>)
            n233 = control-ref of="_IconSearchText"() -> (w500:refnum<vi>)
            n234 = control-ref of="_Manage"() -> (w499:refnum<vi>)
            n235 = control-ref of="_Folders"() -> (w498:refnum<vi>)
            n236 = control-ref of="Icons"() -> (w497:refnum<vi>)
            n237 = Build Array(w501, w500, w499, w498, w497) -> (w496:refnum<vi>[])
            n238 = for {
              tunnel: w496 -> [w503] mode=indexing
              n239 = property class="Ctl"(reference=w503, "Visible"=TRUE) -> ()  [unwired: 1 in, 2 out]
            }
            n240 = property on="_MethodIcons" class="Bool"("Visible"=FALSE) -> ()  [unwired: 2 in, 2 out]
          }
          event "_Cancel": Value Change {
            n241 = event-data() -> ()  [unwired: 1 in, 1 out]
            n242 = Bundle By Name(cluster=w507, "Cancelled"="_Cancel") -> (w505:T5)
          }
          event "_RenameVI": Value Change {
            n243 = event-data() -> ()  [unwired: 1 in, 1 out]
            n244 = Unbundle By Name(w512) -> ("NewName"=w511:string, "ClassInfos"=w510:T19, "Selected"=w509:i32[])
            n245 = for {
              tunnel: w510 -> [w519]
              tunnel: w509 -> [w518] mode=indexing
              tunnel: [w516] -> w508 mode=indexing
              n246 = Index Array(array=w519, index=w518) -> (element=w517:T7)
              n247 = Unbundle By Name(w517) -> ("VI-Path"=w516:path)
            }
            n248 = Bundle By Name(cluster=w515, "RenameOption.NewVIName"=w511, "RenameOption.VIs"=w508) -> (w513:T5)
          }
          event "_IconSearchText": Value Change {
            n249 = event-data() -> ()  [unwired: 1 in, 1 out]
          }
          event "Icons", "DragIcon": Mouse Move {
            n250 = event-data() -> ("Coords"=w525:T3)  [unwired: 1 in]
            n251 = Unbundle By Name(w526) -> ("DraggingIcon"=w527:bool)
            n252 = case shown="False" w527 {
              tunnel: w524 -> [w540 w558]
              tunnel: [w539 w558] -> w523
              tunnel: [w537 "Idle" ("t")] -> w522
              tunnel: w525 -> [w535 _]
              tunnel: w526 -> [w532 _]
              frame False {
                n253 = Unbundle By Name(w532) -> ("IconPos"=w541:T23)
                n254 = property on="Icons" class="Pict"() -> ("Position"=w536:T13)  [unwired: 2 in, 2 out]
                n255 = property on="Icons" class="Pict"() -> ("Origin"=w531:T14)  [unwired: 2 in, 2 out]
                n256 = Subtract(x=w535, y=w536) -> (x-y=w530:T3)
                n257 = Add(x=w531, y=w530) -> (x+y=w529:T3)
                n258 = for {
                  tunnel: w541 -> [w551] mode=indexing
                  tunnel: w529 -> [w553]
                  tunnel: [w543] -> w538
                  tunnel: [w542] -> w534
                  i -> [w542]
                  stop <- w543 stop-if-true
                  n259 = Unbundle(w551) -> ("left"=w550:i16, "top"=w546:i16, "right"=w549:i16, "bottom"=w548:i16)
                  n260 = Unbundle(w553) -> ("Horizontal"=w552:i32, "Vertical"=w547:i32)
                  n261 = In Range and Coerce(upper limit=w549, x=w552, lower limit=w550) -> (In Range?=w544:bool)  [unwired: 1 out]
                  n262 = In Range and Coerce(upper limit=w548, x=w547, lower limit=w546) -> (In Range?=w545:bool)  [unwired: 1 out]
                  n263 = And(x=w544, y=w545) -> (x .and. y?=w543:bool)
                }
                n264 = Select(t=w534, s=w538, f=-1) -> (s? t:f=w528:i32)
                n265 = case shown="True" w538 {
                  tunnel: ["Idle" ("t") "ShowDragIcon" ("t")] -> w537
                  frame False {
                    n266 = property on="DragIcon" class="Pict"("Visible"=FALSE) -> ()  [unwired: 2 in, 2 out]
                  }
                  frame True {
                  }
                }
                n267 = Bundle By Name(cluster=w540, "IconSelected"=w528) -> (w539:T5)
              }
              frame True {
              }
            }
          }
          event Key Down? {
            (unwired) TRUE
            n268 = event-data() -> ("VKey"=w566:T24, "PlatMods"=w565:T25)  [unwired: 1 in, 3 out]
            n269 = property on="_FontCompression" class="Enum (strict)"() -> ("Key Focus"=w569:bool)  [unwired: 2 in, 2 out]
            n270 = property on="_MethodIconName" class="Str"() -> ("Key Focus"=w572:bool)  [unwired: 2 in, 2 out]
            n271 = property on="NewName" class="Str"() -> ("Key Focus"=w559:bool)  [unwired: 2 in, 2 out]
            n272 = property on="_TextAlignment" class="Ring (strict)"() -> ("Key Focus"=w571:bool)  [unwired: 2 in, 2 out]
            n273 = property on="_IconSize" class="Ring (strict)"() -> ("Key Focus"=w570:bool)  [unwired: 2 in, 2 out]
            n274 = Compound Arithmetic op=AND(invert w569, invert w570, invert w571, invert w572, invert w559) -> (w573:bool)
            n275 = Unbundle By Name(w560) -> ("Offset.X"=w568:i32, "Offset.Y"=w567:i32)
            n276 = Unbundle By Name(w565) -> ("Ctrl"=w574:bool)
            n277 = Or(x=w574, y=w573) -> (x .or. y?=w575:bool)
            n278 = case shown="True" w575 {
              tunnel: w562 -> [w577 w581]
              tunnel: [w577 w585] -> w561
              tunnel: w566 -> [_ w584]
              tunnel: w567 -> [_ w578]
              tunnel: w568 -> [_ w579]
              tunnel: ["Idle" w583] -> w563
              tunnel: [_ w582] -> w564
              frame False {
              }
              frame True {
                n279 = Bundle By Name(cluster=w581, "OldOffset.X"=w579, "OldOffset.Y"=w578) -> (w580:T5)
                n280 = case shown="\"Up\"" w584 {
                  tunnel: w580 -> [w592 w594 w596 w603 w610]
                  tunnel: [w591 w594 w595 w602 w609] -> w585
                  tunnel: w578 -> [w590 _ w601 w604 w611]
                  tunnel: w579 -> [w588 _ w597 w608 w615]
                  tunnel: ["Generate icon" "Idle" "Generate icon" "Generate icon" "Generate icon"] -> w583
                  tunnel: [TRUE _ TRUE TRUE TRUE] -> w582
                  frame "Up" {
                    n281 = Decrement(x=w590) -> (x-1=w589:i32)
                    n282 = Bundle By Name(cluster=w592, "Offset.X"=w588, "Offset.Y"=w589) -> (w591:T5)
                  }
                  frame Default {
                  }
                  frame "Down" {
                    n283 = Increment(x=w601) -> (x+1=w598:i32)
                    n284 = Bundle By Name(cluster=w596, "Offset.X"=w597, "Offset.Y"=w598) -> (w595:T5)
                  }
                  frame "Left" {
                    n285 = Decrement(x=w608) -> (x-1=w605:i32)
                    n286 = Bundle By Name(cluster=w603, "Offset.X"=w605, "Offset.Y"=w604) -> (w602:T5)
                  }
                  frame "Right" {
                    n287 = Increment(x=w615) -> (x+1=w612:i32)
                    n288 = Bundle By Name(cluster=w610, "Offset.X"=w612, "Offset.Y"=w611) -> (w609:T5)
                  }
                }
              }
            }
            n289 = event-data("Discard?"=w564) -> ()  [unwired: 1 in, 1 out]
          }
          event "_Folders": Value Change {
            n290 = event-data() -> ()  [unwired: 1 in, 1 out]
          }
          event "_Manage": Value Change {
            n291 = event-data() -> ()  [unwired: 1 in, 1 out]
            n292 = call <resource>:"GDSLvIcon_ManageIconFolderDialog.vi"() -> ("Cancelled"=w619:bool)  [unwired: 10 in, 1 out]
            n293 = Select(t="Idle", s=w619, f="UpdateIconFolderList" ("y")) -> (s? t:f=w618:string)
          }
          event "_MethodIconName", "_TextAlignment", "_FontCompression", "_HideHeader", "_IconSize", "_CapitalOnly": Value Change {
            n294 = event-data() -> ()  [unwired: 1 in, 1 out]
          }
          event "_IconPreview": Mouse Down {
            w642 = 4 ("y")
            n295 = event-data() -> ("Coords"=w629:T3)  [unwired: 1 in]
            n296 = property on="_IconPreview" class="Pict"() -> ("Mouse"=w638:T26)  [unwired: 2 in, 2 out]
            n297 = Unbundle By Name(w638) -> ("Mouse Position.X"=w641:i32, "Mouse Position.Y"=w639:i32)
            n298 = Unbundle By Name(w625) -> ("IconDropped"=w630:i32, "TextBounds"=w631:T21)
            n299 = Unbundle(w631) -> ("FirstRow"=w633:i32, "FirstColumn"=w634:i32, "LastRow"=w632:i32, "LastColumn"=w637:i32)
            n300 = Divide(x=w641, y=w642) -> (x/y=w643:dbl)
            n301 = Divide(x=w639, y=w642) -> (x/y=w640:dbl)
            n302 = In Range and Coerce(upper limit=w632, x=w640, lower limit=w633) -> (In Range?=w635:bool)  [unwired: 1 out]
            n303 = In Range and Coerce(upper limit=w637, x=w643, lower limit=w634) -> (In Range?=w636:bool)  [unwired: 1 out]
            n304 = And(x=w635, y=w636) -> (x .and. y?=w644:bool)
            n305 = case shown="False" w644 {
              tunnel: w628 -> [w649 w680]
              tunnel: [w648 w677] -> w627
              tunnel: [w647 "Idle" ("y")] -> w626
              tunnel: w629 -> [w646 w671]
              tunnel: w630 -> [w645 _]
              tunnel: w625 -> [_ w675]
              frame False {
                n306 = case shown="0.." w645 {
                  selector: w645 -> [_ w652]
                  tunnel: w649 -> [w651 w667]
                  tunnel: [w651 w666] -> w648
                  tunnel: ["Idle" ("y") "ShowDragIcon:UpdateIcon" ("y")] -> w647
                  tunnel: w646 -> [_ w653]
                  frame Default {
                  }
                  frame 0.. {
                    n307 = property on="DragIcon" class="Pict"() -> ("Draw Area Size"=w664:T22)  [unwired: 2 in, 2 out]
                    n308 = Divide(x=w664, y=2) -> (x/y=w662:cluster{"Width":dbl, "Height":dbl})
                    n309 = Subtract(x=w653, y=w662) -> (x-y=w656:cluster{dbl, dbl})
                    n310 = property on="_IconPreview" class="Pict"() -> ("Position"=w660:T13)  [unwired: 2 in, 2 out]
                    n311 = property on="DragIcon" class="Pict"("Position"=w656) -> ()  [unwired: 2 in, 2 out]
                    n312 = Add(x=w660, y=T13 {"Left"=0, "Top"=16}) -> (x+y=w659:T13)
                    n313 = Subtract(x=w656, y=w659) -> (x-y=w657:cluster{dbl, dbl})
                    n314 = Divide(x=w657, y=u8 4 ("Disabled")) -> (x/y=w655:cluster{dbl, dbl})
                    n315 = Bundle By Name(cluster=w667, "IconSelected"=w652, "DraggingIcon"=TRUE ("Draging"), "BgIconOffset"=w655) -> (w666:T5)
                  }
                }
              }
              frame True {
                n316 = Unbundle By Name(w675) -> ("Offset.X"=w674:i32, "Offset.Y"=w673:i32)
                n317 = Bundle("X"=w674, "Y"=w673) -> (w669:cluster{"X":i32, "Y":i32})  [unwired: 1 in]
                n318 = Multiply(x=w669, y=4) -> (x*y=w668:cluster{"X":i32, "Y":i32})
                n319 = Subtract(x=w671, y=w668) -> (x-y=w670:T3)
                n320 = Bundle By Name(cluster=w680, "DraggingIcon"=FALSE, "DraggingText"=TRUE, "StartTextDraggingPos"=w670) -> (w677:T5)
              }
            }
          }
          event "_IconPreview": Mouse Up {
            w684 = FALSE ("Draging")
            n321 = event-data() -> ()  [unwired: 1 in, 3 out]
            n322 = Unbundle By Name(w683) -> ("IconSelected"=w685:i32)
            n323 = Bundle By Name(cluster=w682, "IconDropped"=w685, "Moving"=w684, "DraggingIcon"=w684) -> (w681:T5)
            n324 = property on="DragIcon" class="Pict"("Visible"=w684) -> ()  [unwired: 2 in, 2 out]
          }
          event "_IconPreview": Mouse Enter {
            n325 = event-data() -> ()  [unwired: 1 in, 1 out]
            n326 = Unbundle By Name(w688) -> ("DraggingIcon"=w690:bool, "IconDropped"=w689:i32)
            n327 = case shown="True" w690 {
              tunnel: w687 -> [w693 w694]
              tunnel: [w692 w694] -> w686
              tunnel: w689 -> [w691 _]
              frame False {
                n328 = Bundle By Name(cluster=w693, "IconSelected"=w691) -> (w692:T5)
              }
              frame True {
              }
            }
          }
          event Mouse Up; Mouse Leave {
            w695 = FALSE ("DraggingText")
            n329 = event-data() -> ()  [unwired: 1 in, 4 out]
            n330 = Bundle By Name(cluster=w697, "DraggingText"=w695, "DraggingIcon"=w695) -> (w696:T5)
            n331 = property on="DragIcon" class="Pict"("Visible"=w695) -> ()  [unwired: 2 in, 2 out]
          }
          event Mouse Move {
            n332 = event-data() -> ("Coords"=w700:T3)  [unwired: 1 in]
            n333 = Unbundle By Name(w701) -> ("StartTextDraggingPos"=w705:T3)
            n334 = Unbundle By Name(w701) -> ("DraggingText"=w704:bool, "DraggingIcon"=w703:bool)
            n335 = case shown="False" w703 {
              tunnel: w699 -> [w711 w736]
              tunnel: [w710 w735] -> w698
              tunnel: w700 -> [w707 w731]
              tunnel: w701 -> [w706 _]
              tunnel: [w709 "UpdateIcon" ("y")] -> w702
              tunnel: w704 -> [w712 _]
              tunnel: w705 -> [w708 _]
              frame False {
                n336 = case shown="False" w712 {
                  tunnel: w711 -> [w714 w729]
                  tunnel: [w714 w728] -> w710
                  tunnel: [_ "Generate icon"] -> w709
                  tunnel: w708 -> [_ w725]
                  tunnel: w707 -> [_ w726]
                  tunnel: w706 -> [_ w724]
                  frame False {
                    n337 = property on="NewName" class="Str"() -> ("Key Focus"=w713:bool)  [unwired: 2 in, 2 out]
                    n338 = case shown="False" w713 {
                      selector: w713 -> [w715 _]
                      frame False {
                        n339 = property on="Ballon" class="Clust (strict)"("Visible"=w715) -> ()  [unwired: 2 in, 2 out]
                      }
                      frame True {
                      }
                    }
                  }
                  frame True {
                    n340 = Subtract(x=w726, y=w725) -> (x-y=w721:T3)
                    n341 = Unbundle By Name(w724) -> ("Offset.X"=w719:i32, "Offset.Y"=w718:i32)
                    n342 = Divide(x=w721, y=u8 4 ("f")) -> (x/y=w720:cluster{"Horizontal":dbl, "Vertical":dbl})
                    n343 = Unbundle By Name(w720) -> ("Horizontal"=w717:dbl, "Vertical"=w716:dbl)
                    n344 = Bundle By Name(cluster=w729, "OldOffset.X"=w719, "OldOffset.Y"=w718) -> (w723:T5)
                    n345 = Bundle By Name(cluster=w723, "Offset.X"=w717, "Offset.Y"=w716) -> (w728:T5)
                  }
                }
              }
              frame True {
                n346 = property on="DragIcon" class="Pict"() -> ("Draw Area Size"=w741:T22)  [unwired: 2 in, 2 out]
                n347 = property on="_IconPreview" class="Pict"() -> ("Position"=w739:T13)  [unwired: 2 in, 2 out]
                n348 = Divide(x=w741, y=2.0 ("Waveform Chart")) -> (x/y=w742:cluster{"Width":dbl, "Height":dbl})
                n349 = Add(x=w739, y=T13 {"Left"=0, "Top"=16}) -> (x+y=w738:T13)
                n350 = Subtract(x=w731, y=w742) -> (x-y=w730:cluster{dbl, dbl})
                n351 = Subtract(x=w730, y=w738) -> (x-y=w733:cluster{dbl, dbl})
                n352 = property on="DragIcon" class="Pict"("Position"=w730) -> ()  [unwired: 2 in, 2 out]
                n353 = Divide(x=w733, y=u8 4 ("Disabled")) -> (x/y=w732:cluster{dbl, dbl})
                n354 = Bundle By Name(cluster=w736, "BgIconOffset"=w732) -> (w735:T5)
              }
            }
          }
          event "Ballon", "Tree": Mouse Enter {
            n355 = event-data() -> ()  [unwired: 1 in, 4 out]
            n356 = Unbundle By Name(w747) -> ("StartTime"=w746:i32)
            n357 = Tick Count (ms)() -> (millisecond timer value=w745:u32)
            n358 = Subtract(x=w745, y=w746) -> (x-y=w744:u32)
            n359 = case shown="3000.." w744 {
              frame 0, Default {
              }
              frame 3000.. {
                n360 = property on="Ballon" class="Clust (strict)"("Visible"=FALSE) -> ()  [unwired: 2 in, 2 out]
              }
            }
          }
          event "Tree": Double Click {
            n361 = event-data() -> ("Tag"=w750:string)  [unwired: 1 in]
            n362 = Match Pattern(string=w750, regular expression=":VI$") -> (offset past match=w755:i32)  [unwired: 1 in, 3 out]
            n363 = case shown="0, Default" w755 {
              tunnel: [w758 "Idle"] -> w754
              tunnel: [w766 w783] -> w753
              tunnel: w752 -> [w767 w783]
              tunnel: w751 -> [w765 _]
              tunnel: w750 -> [w763 _]
              frame 0, Default {
                n364 = Unbundle By Name(w765) -> ("ClassIndex"=w760:i32, "Selected"=w762:i32[], "TreeTags"=w764:string[])
                n365 = Search 1D Array(1D array=w764, element=w763) -> (index of element=w757:i32)  [unwired: 1 in]
                n366 = Search 1D Array(1D array=w762, element=w757) -> (index of element=w761:i32)  [unwired: 1 in]
                n367 = Equal?(x=w760, y=w757) -> (x = y?=w759:bool)
                n368 = case shown="False" w759 {
                  tunnel: w767 -> [w774 w782]
                  tunnel: [w773 w782] -> w766
                  tunnel: w762 -> [w772 _]
                  tunnel: w757 -> [w771 _]
                  tunnel: w761 -> [w770 _]
                  tunnel: ["UpdateClassList" "Idle"] -> w758
                  frame False {
                    n369 = case shown="0, Default" w770 {
                      selector: w770 -> [w776 _]
                      tunnel: w772 -> [w777 w780]
                      tunnel: w771 -> [_ w779]
                      tunnel: [w775 w778] -> w769
                      frame 0, Default {
                        n370 = Delete From Array(array=w777, index=w776) -> (array with subset deleted=w775:i32[])  [unwired: 1 in, 1 out]
                      }
                      frame -1 {
                        n371 = Build Array (concatenate)(w780, w779) -> (w778:i32[])
                      }
                    }
                    n372 = Bundle By Name(cluster=w774, "Selected"=w769) -> (w773:T5)
                  }
                  frame True {
                  }
                }
              }
              frame -1 {
              }
            }
          }
          event Panel Close? {
            w785 = TRUE ("Discard?")
            n373 = event-data() -> ()  [unwired: 1 in, 1 out]
            n374 = Bundle By Name(cluster=w787, "Cancelled"=w785) -> (w786:T5)
            n375 = event-data("Discard?"=w785) -> ()  [unwired: 1 in, 1 out]
          }
          event "FloodFillMask": Value Change {
            n376 = event-data() -> ()  [unwired: 1 in, 1 out]
            n377 = Unbundle By Name(w790) -> ("BgIcon"=w794:u8[][])
            n378 = call <resource>:"GDSIconEditor_CreateImageMask.vi"("Flood Fill"="FloodFillMask", "8-bit pixmap"=w794) -> ("Array"=w795:u8[])
            n379 = Bundle By Name(cluster=w793, "BgIconMask"=w795) -> (w792:T5)
          }
          event "Help": Value Change {
            n380 = event-data() -> ()  [unwired: 1 in, 6 out]
            n381 = call <resource>:"GOOP_HelpMain.vi"() -> ()  [unwired: 12 in]
          }
          event "_ShowContextHelp": Value Change {
            n382 = event-data() -> ("NewVal"=w798:bool)  [unwired: 1 in]
            n383 = Control Help Window(1:w798) -> ()  [unwired: 1 in]
          }
        }
      }
      frame "GetImageData" {
        # "Create White mask Color, When Mouse Down"
        n384 = Unbundle By Name(w801) -> ("Icons"=w804:T4[], "IconSelected"=w805:i32)
        n385 = Index Array(array=w804, index=w805) -> (element=w808:T4)
        n386 = call <resource>:"GDSIconEditor_ImageDataTo8Bit.vi"("image data"=w808) -> ("NoMaskFound"=w802:bool, "8-bit pixmap"=w809:u8[][], "mask"=w806:u8[])  [unwired: 7 in, 1 out]
        n387 = property on="FloodFillMask" class="Bool (strict)"("Visible"=w802) -> ()  [unwired: 2 in, 2 out]
        n388 = case shown="True" w802 {
          tunnel: w809 -> [_ w814]
          tunnel: w806 -> [w811 _]
          tunnel: [w811 w813] -> w807
          frame False {
          }
          frame True {
            n389 = local read "FloodFillMask"() -> (w812:bool)
            n390 = call <resource>:"GDSIconEditor_CreateImageMask.vi"("Flood Fill"=w812, "8-bit pixmap"=w814) -> ("Array"=w813:u8[])
          }
        }
        n391 = call <vilib>:"Draw Flattened Pixmap.vi"("image data"=w808) -> ("new picture"=→"DragIcon":picture)  [unwired: 8 in]
        n392 = Bundle By Name(cluster=w801, "BgIcon"=w809, "BgIconMask"=w807) -> (w800:T5)
      }
      frame "ShowDragIcon", "ShowDragIcon:UpdateIcon" {
        w829 = 2.0 ("Waveform Chart")
        w840 = 4 ("x")
        n393 = Unbundle By Name(w817) -> ("IconNames"=w854:string[], "Icons"=w818:T4[], "IconSelected"=w855:i32, "IconPos"=w821:T23)
        n394 = Index Array(array=w854, index=w855) -> ()  [unwired: 1 out]
        n395 = Index Array(array=w818, index=w855) -> (element=w856:T4)
        n396 = Index Array(array=w821, index=w855) -> (element=w822:T27)
        n397 = Unbundle By Name(w822) -> ("left"=w823:i16, "top"=w827:i16, "right"=w824:i16, "bottom"=w826:i16)
        n398 = call <resource>:"GDSIconEditor_ShrinkImage.vi"("image data"=w856) -> ("image subset"=w857:T4)  [unwired: 9 in]
        n399 = Unbundle By Name(w857) -> ("Rectangle.right"=w847:i16, "Rectangle.bottom"=w846:i16)
        n400 = call <vilib>:"Draw Flattened Pixmap.vi"("image data"=w857) -> ("new picture"=w838:picture)  [unwired: 8 in]
        n401 = property on="Icons" class="Pict"() -> ("Position"=w852:T13)  [unwired: 2 in, 2 out]
        n402 = property on="Icons" class="Pict"() -> ("Origin"=w851:T14)  [unwired: 2 in, 2 out]
        n403 = Add(x=w827, y=w826) -> (x+y=w828:i16)
        n404 = Add(x=w823, y=w824) -> (x+y=w825:i16)
        n405 = Divide(x=w828, y=w829) -> (x/y=w831:dbl)
        n406 = Divide(x=w825, y=w829) -> (x/y=w830:dbl)
        n407 = Subtract(x=w852, y=w851) -> (x-y=w853:T13)
        n408 = Bundle("right"=w847, "bottom"=w846) -> (w839:cluster{"right":i16, "bottom":i16})  [unwired: 1 in]
        n409 = Bundle(w830, w831) -> (w832:cluster{dbl, dbl})  [unwired: 1 in]
        n410 = Increment(x=w839) -> (x+1=w820:cluster{"right":i16, "bottom":i16})
        n411 = Add(x=w832, y=w853) -> (x+y=w833:cluster{dbl, dbl})
        n412 = Divide(x=w820, y=2.0 ("Waveform Chart")) -> (x/y=w841:cluster{"right":dbl, "bottom":dbl})
        n413 = Multiply(x=w840, y=w841) -> (x*y=w842:cluster{"right":dbl, "bottom":dbl})
        n414 = Subtract(x=w833, y=w842) -> (x-y=w849:cluster{dbl, dbl})
        n415 = Multiply(x=w840, y=w847) -> (x*y=w836:i32)
        n416 = Multiply(x=w840, y=w846) -> (x*y=w837:i32)
        n417 = Equal?(x=w816, y="ShowDragIcon:UpdateIcon") -> (x = y?=w850:bool)
        n418 = Bundle(w836, w837) -> (w835:cluster{i32, i32})  [unwired: 1 in]
        n419 = Select(t="UpdateIcon", s=w850, f="Idle" ("y")) -> (s? t:f=w815:string)
        n420 = property on="DragIcon" class="Pict"("Draw Area Size"=w835, "Value"=w838, "Visible"=TRUE) -> (error out=w848:errorcluster)  [unwired: 2 in, 1 out]
        n421 = case shown="False" w850 {
          tunnel: w848 -> [w860 _]
          tunnel: w849 -> [w859 _]
          frame False {
            n422 = property on="DragIcon" class="Pict"(error in=w860, "Position"=w859) -> ()  [unwired: 1 in, 2 out]
          }
          frame True {
          }
        }
      }
      frame "UpdateIconFolderList" {
        n423 = VI Library() -> (path=w893:path)
        n424 = call <resource>:"GOOP_GetGDSConfigFolder.vi"() -> ("GDSFolderPath"=w866:path)
        n425 = call <vilib>:"Set Busy.vi"("error in (no error)"=w865) -> ("error out"=w864:errorcluster)  [unwired: 9 in, 1 out]
        n426 = Strip Path(path=w893) -> (stripped path=w881:path)  [unwired: 1 out]
        n427 = call <resource>:"GOOP_GetProviderIniFilePath.vi"() -> ("ProviderMainFolder"=w905:path)  [unwired: 10 in, 1 out]
        n428 = Build Path(base path=w866, name or relative path="IconFolder.txt") -> (appended path=w874:path)
        n429 = Read from Text File(file (use dialog)=w874) -> (text=w868:string)  [unwired: 3 in, 3 out]
        n430 = Build Path(base path=w881, name or relative path="resource") -> (appended path=w892:path)
        n431 = call <vilib>:"Dflt Data Dir.vi"() -> ("App:Default Data Directory"=w885:path)
        n432 = call <vilib>:"Trim Whitespace.vi"("string"=w868) -> ("trimmed string"=w878:string)  [unwired: 1 in]
        n433 = Build Path(base path=w892, name or relative path="Framework") -> (appended path=w891:path)
        n434 = Spreadsheet String To Array(delimiter (Tab)="\n", format string="%s", spreadsheet string=w878, array type (2D Dbl)=string[] []) -> (array=w899:string[])
        n435 = Build Path(base path=w885, name or relative path="Glyphs") -> (appended path=w884:path)
        n436 = Build Path(base path=w891, name or relative path="Providers") -> (appended path=w882:path)
        n437 = Build Path(base path=w882, name or relative path="Icons") -> (appended path=w897:path)
        n438 = Build Path(base path=w905, name or relative path="Glyphs") -> (appended path=w903:path)
        n439 = Build Path(base path=w905, name or relative path="Icons") -> (appended path=w906:path)
        n440 = Path To String(path=w897) -> (string=w895:string)
        n441 = Path To String(path=w903) -> (string=w896:string)
        n442 = Path To String(path=w906) -> (string=w907:string)
        n443 = Path To String(path=w884) -> (string=w894:string)
        n444 = Build Array(w894, w895, w896, w907) -> (w898:string[])
        n445 = Build Array (concatenate)(w898, w899) -> (w900:string[])
        n446 = for {
          tunnel: w900 -> [w909] mode=indexing
          tunnel: [w912] -> w902 mode=indexing
          tunnel: [w908] -> w901 mode=indexing
          n447 = String To Path(string=w909) -> (path=w912:path)
          n448 = String Length(string=w909) -> (length=w910:i32)
          n449 = Subtract(x=w910, y=38) -> (x-y=w911:i32)
          n450 = case shown="1.." w911 {
            selector: w911 -> [_ w921]
            tunnel: w910 -> [_ _]
            tunnel: w909 -> [w914 w919]
            tunnel: [w914 w916] -> w908
            frame 0, Default {
            }
            frame 1.. {
              n451 = Add(x=w921, y=3) -> (x+y=w918:i32)
              n452 = String Subset(string=w919, offset (0)=w918) -> (substring=w917:string)  [unwired: 1 in]
              n453 = Concatenate Strings("..." ("string"), w917) -> (w916:string)
            }
          }
        }
        n454 = for {
          tunnel: w902 -> [w926] mode=indexing
          shift-right: [w931] -> w877
          shift-left: path[] [] -> [w927]
          shift-right: [w930] -> w880
          shift-left: string[] [] -> [w929]
          tunnel: w901 -> [w928] mode=indexing
          n455 = Empty String/Path?(string/path=w926) -> (empty?=w924:bool)
          n456 = Search 1D Array(1D array=w927, element=w926) -> (index of element=w925:i32)  [unwired: 1 in]
          n457 = Greater Or Equal To 0?(x=w925) -> (x >= 0?=w923:bool)
          n458 = Or(x=w924, y=w923) -> (x .or. y?=w922:bool)
          n459 = case shown="False" w922 {
            tunnel: w926 -> [w935 _]
            tunnel: w927 -> [w938 w948]
            tunnel: [w937 w948] -> w931
            tunnel: w929 -> [w933 w947]
            tunnel: [w934 w947] -> w930
            tunnel: w928 -> [w932 _]
            frame False {
              n460 = call <vilib>:"Check if File or Folder Exists.vi"("path"=w935) -> ("file or folder exists?"=w936:bool)  [unwired: 8 in, 2 out]
              n461 = case shown="True" w936 {
                tunnel: w938 -> [w940 w946]
                tunnel: [w940 w945] -> w937
                tunnel: w935 -> [_ w944]
                tunnel: w933 -> [w939 w942]
                tunnel: [w939 w943] -> w934
                tunnel: w932 -> [_ w941]
                frame False {
                }
                frame True {
                  n462 = Build Array (concatenate)(w946, w944) -> (w945:path[])
                  n463 = Build Array (concatenate)(w942, w941) -> (w943:string[])
                }
              }
            }
            frame True {
            }
          }
        }
        n464 = Build Array (concatenate)("<All icons>" ("y"), w880) -> (w873:string[])
        n465 = property on="_Folders" class="Ring (strict)"("Strings []"=w873, "Value"=1) -> ()  [unwired: 2 in, 2 out]
        n466 = Bundle By Name(cluster=w862, "Folders"=w877) -> (w861:T5)
      }
      frame "ReadIcons" {
        (unwired) "" ("Name")
        n467 = local read "_Folders"() -> (w951:u16)
        n468 = Unbundle By Name(w953) -> ("Folders"=w954:path[])
        n469 = case shown="Default" w951 {
          tunnel: w954 -> [w961 w966]
          tunnel: w951 -> [_ w965]
          tunnel: [w961 w962] -> w955
          frame 0 {
            (unwired) 0 ("index")
          }
          frame Default {
            n470 = Decrement(x=w965) -> (x-1=w964:u16)
            n471 = Index Array(array=w966, index=w964) -> (element=w963:path)
            n472 = Build Array(w963) -> (w962:path[])
          }
        }
        n473 = call <vilib>:"Set Busy.vi"("error in (no error)"=w950) -> ("error out"=w956:errorcluster)  [unwired: 9 in, 1 out]
        n474 = for {
          tunnel: w955 -> [w971] mode=indexing
          shift-right: [w967] -> w958
          shift-left: cluster{i32, "path out":path}[] [] -> [w968]
          shift-right: [w972] -> w949
          shift-left: w956 -> [w969]
          n475 = call <vilib>:"Check if File or Folder Exists.vi"("path"=w971) -> ("file or folder exists?"=w970:bool)  [unwired: 8 in, 2 out]
          n476 = case shown="True" w970 {
            tunnel: [w974 w980] -> w972
            tunnel: w969 -> [w974 w979]
            tunnel: w971 -> [_ w978]
            tunnel: w968 -> [w973 w975]
            tunnel: [w973 w977] -> w967
            frame False {
            }
            frame True {
              n477 = call <vilib>:"Recursive File List.vi"("pattern"="*.png", "error in (no error)"=w979, "Folder Path"=w978) -> ("error out"=w982:errorcluster, "All Files in Dir"=w983:path[])  [unwired: 4 in, 3 out]
              n478 = for {
                tunnel: w983 -> [w991] mode=indexing
                tunnel: [w989] -> w976 mode=indexing
                shift-right: [w988] -> w980
                shift-left: w982 -> [w992]
                n479 = File/Directory Info(path=w991, error in=w992) -> (path out=w990:path, size=w987:i64, error out=w988:errorcluster)  [unwired: 4 out]
                n480 = Divide(x=w987, y=i64 100) -> (x/y=w985:dbl)
                n481 = To Long Integer(number=w985) -> (32bit integer=w984:i32)
                n482 = Bundle(w984, "path out"=w990) -> (w989:cluster{i32, "path out":path})  [unwired: 1 in]
              }
              n483 = Build Array (concatenate)(w975, w976) -> (w977:cluster{i32, "path out":path}[])
            }
          }
        }
        n484 = Sort 1D Array(array=w958) -> (sorted array=w959:cluster{i32, "path out":path}[])
        n485 = Bundle By Name(cluster=w953, "IconPaths"=w959) -> (w952:T5)
      }
      frame "DrawIcons", "DrawIcons:NoBusy" {
        w1005 = 0  # IconsPerRow
        w1001 = 10  # Border
        w1003 = 15  # Gap
        # "Y"
        # "X"
        n486 = Unbundle By Name(w998) -> ("IconPaths"=w1015:cluster{i32, "path out":path}[])
        n487 = case shown="\"DrawIcons:NoBusy\"" w993 {
          tunnel: w1000 -> [w1019 w1021]
          tunnel: [w1019 w1020] -> w1016
          frame "DrawIcons:NoBusy" {
          }
          frame Default {
            n488 = call <vilib>:"Set Busy.vi"("error in (no error)"=w1021) -> ("error out"=w1020:errorcluster)  [unwired: 9 in, 1 out]
          }
        }
        n489 = property on="Icons" class="Pict"() -> ("Draw Area Size"=w1008:T22)  [unwired: 2 in, 2 out]
        n490 = local read "_IconSearchText"() -> (w994:string)
        n491 = Unbundle By Name(w1008) -> ("Width"=w1002:u32)
        n492 = property on="Icons" class="Pict"("Origin"=T14 {"Horizontal"=0, "Vertical"=0}) -> ()  [unwired: 2 in, 2 out]
        n493 = call <vilib>:"Trim Whitespace.vi"("string"=w994) -> ("trimmed string"=w1017:string)  [unwired: 1 in]
        n494 = for {
          shift-right: [w1050] -> w999
          shift-left: w1016 -> [w1033]
          shift-right: [w1037] -> _
          shift-left: w1001 -> [w1045]
          shift-right: [w1048] -> w995
          shift-left: picture data[5B] ("new picture") -> [w1049]
          shift-right: [w1046] -> w1009
          shift-left: T4[] [] -> [w1047]
          shift-right: [w1038] -> _
          shift-left: w1005 -> [w1039]
          shift-right: [w1036] -> _
          shift-left: w1001 -> [w1040]
          shift-right: [w1041] -> _
          shift-left: TRUE -> [w1044]
          tunnel: w1003 -> [w1043]
          tunnel: w1002 -> [w1042]
          tunnel: w1001 -> [w1035]
          tunnel: w1015 -> [w1034] mode=indexing
          shift-right: [w1032] -> w1011
          shift-left: cluster{i32, i32, i32, i32}[] [] -> [w1031]
          shift-right: [w1029] -> w1014
          shift-left: string[] [] -> [w1030]
          tunnel: w1017 -> [w1028]
          n495 = Unbundle(w1034) -> (w1026:i32, "path out"=w1027:path)
          n496 = case shown="\"\"" w1028 {
            selector: w1028 -> [w1056 _]
            tunnel: w1027 -> [w1057 _]
            tunnel: [w1051 TRUE] -> w1023
            frame Default {
              n497 = To Lower Case(string=w1056) -> (all lower case string=w1053:string)
              n498 = call <vilib>:"Get File Extension.vi"("file"=w1057) -> ("filename without extension"=w1055:string)  [unwired: 6 in, 4 out]
              n499 = To Lower Case(string=w1055) -> (all lower case string=w1054:string)
              n500 = Match Pattern(string=w1054, regular expression=w1053) -> (offset past match=w1052:i32)  [unwired: 1 in, 3 out]
              n501 = Greater Or Equal To 0?(x=w1052) -> (x >= 0?=w1051:bool)
            }
            frame "" {
            }
          }
          n502 = Less Or Equal?(x=w1026, y=50) -> (x <= y?=w1024:bool)
          n503 = And(x=w1023, y=w1024) -> (x .and. y?=w1022:bool)
          n504 = case shown="True" w1022 {
            tunnel: w1027 -> [_ w1071]
            tunnel: w1033 -> [w1067 w1100]
            tunnel: [w1067 w1099] -> w1050
            tunnel: w1049 -> [w1066 w1098]
            tunnel: [w1066 w1077] -> w1048
            tunnel: w1047 -> [w1065 w1083]
            tunnel: [w1065 w1097] -> w1046
            tunnel: w1045 -> [w1063 w1080]
            tunnel: w1044 -> [w1061 w1096]
            tunnel: w1043 -> [_ w1082]
            tunnel: w1042 -> [_ w1093]
            tunnel: [w1061 w1092] -> w1041
            tunnel: w1040 -> [w1062 w1087]
            tunnel: w1039 -> [w1064 w1086]
            tunnel: [w1064 w1085] -> w1038
            tunnel: [w1063 w1075] -> w1037
            tunnel: [w1062 w1079] -> w1036
            tunnel: w1035 -> [_ w1081]
            tunnel: w1031 -> [w1060 w1074]
            tunnel: [w1060 w1073] -> w1032
            tunnel: w1030 -> [w1059 w1069]
            tunnel: [w1059 w1070] -> w1029
            frame False {
            }
            frame True {
              # "Place This Icon on a new row"
              n505 = call <vilib>:"Read PNG File.vi"("error in (no error)"=w1100, "path to PNG file"=w1071) -> ("error out"=w1099:errorcluster, "image data"=w1091:T4)  [unwired: 7 in, 1 out]
              n506 = Unbundle By Name(w1091) -> ("Rectangle"=w1090:T27)
              n507 = Unbundle By Name(w1091) -> ("Rectangle.right"=w1078:i16)
              n508 = Select(t=0, s=w1096, f=w1082) -> (s? t:f=w1095:i32)
              n509 = Add(x=w1095, y=w1080) -> (x+y=w1088:i32)
              n510 = Strip Path(path=w1071) -> (name=w1068:string)  [unwired: 1 out]
              n511 = Add(x=w1088, y=w1078) -> (x+y=w1084:i32)
              n512 = Greater?(x=w1084, y=w1093) -> (0:w1092:bool)
              n513 = Build Array (concatenate)(w1083, w1091) -> (w1097:T4[])
              n514 = case shown="True" w1092 {
                tunnel: [w1105 w1111] -> w1089
                tunnel: w1088 -> [w1102 _]
                tunnel: w1087 -> [w1101 w1106]
                tunnel: w1086 -> [w1104 w1114]
                tunnel: [w1103 1] -> w1085
                tunnel: w1083 -> [_ w1115]
                tunnel: w1082 -> [_ w1109]
                tunnel: w1081 -> [_ w1108]
                tunnel: w1080 -> [_ _]
                tunnel: [w1101 w1107] -> w1079
                tunnel: w1078 -> [_ _]
                frame False {
                  n515 = Bundle(w1102, "Border"=w1101, w1102, "Border"=w1101) -> (w1105:cluster{i32, "Border":i32, i32, "Border":i32})  [unwired: 1 in]
                  n516 = Increment(x=w1104) -> (x+1=w1103:i32)
                }
                frame True {
                  n517 = Delete From Array(array=w1115, length=w1114) -> (deleted portion=w1113:T4[])  [unwired: 1 in, 1 out]
                  n518 = for {
                    tunnel: w1113 -> [w1118] mode=indexing
                    tunnel: [w1117] -> w1112 mode=indexing
                    n519 = Unbundle By Name(w1118) -> ("Rectangle.bottom"=w1117:i16)
                  }
                  n520 = Array Max & Min(array=w1112) -> (max value=w1110:i16)  [unwired: 3 out]
                  n521 = Compound Arithmetic op=ADD(w1106, w1109, w1110) -> (w1107:i32)
                  n522 = Bundle("Border"=w1108, w1107, "Border"=w1108, w1107) -> (w1111:cluster{"Border":i32, i32, "Border":i32, i32})  [unwired: 1 in]
                }
              }
              n523 = Add(x=w1089, y=w1090) -> (x+y=w1072:cluster{i32, i32, i32, i32})
              n524 = Bundle By Name(cluster=w1091, "Rectangle"=w1072) -> (w1076:T4)
              n525 = Build Array (concatenate)(w1074, w1072) -> (w1073:cluster{i32, i32, i32, i32}[])
              n526 = Build Array (concatenate)(w1069, w1068) -> (w1070:string[])
              n527 = Unbundle By Name(w1076) -> ("Rectangle.right"=w1075:i16)
              n528 = call <vilib>:"Draw Flattened Pixmap.vi"("image data"=w1076, "picture"=w1098) -> ("new picture"=w1077:picture)  [unwired: 7 in]
            }
          }
        }
        "Icons" <- w995
        n529 = property on="DragIcon" class="Pict"("Visible"=FALSE) -> ()  [unwired: 2 in, 2 out]
        n530 = Bundle By Name(cluster=w998, "Icons"=w1009, "IconPos"=w1011, "IconNames"=w1014) -> (w997:T5)
        n531 = call <vilib>:"Unset Busy.vi"("error in (no error)"=w999) -> ()  [unwired: 10 in, 1 out]
      }
      frame "PlaceIcon" {
        n532 = Unbundle By Name(w1121) -> ("Icons"=w1122:T4[], "IconSelected"=w1123:i32)
        n533 = Index Array(array=w1122, index=w1123) -> (element=w1126:T4)
        n534 = call <resource>:"GDSIconEditor_ShrinkImage.vi"("image data"=w1126) -> ("image subset"=w1127:T4)  [unwired: 9 in]
        n535 = call <resource>:"GDSIconEditor_ImageDataTo8Bit.vi"("image data"=w1127) -> ("8-bit pixmap"=w1125:u8[][])  [unwired: 7 in, 3 out]
        n536 = Bundle By Name(cluster=w1121, "BgIcon"=w1125, "BgIconOffset"=cluster{"X":i32, "Y":i32} {"X"=0, "Y"=0}) -> (w1120:T5)
      }
      frame "UpdateIcon", "UpdateIcon,Exit" {
        w1146 = T20 {"BgIcon"=[], "BgIconOffset"={"X"=0, "Y"=0}, "BgIconMask"=[], "ColorsOkayforiconToBeOnTopOf"=[]}  # BgIcon
        n537 = Unbundle By Name(w1135) -> ("StartIconSize"=w1153:u16, "StartRow"=w1156:i32, "FrameColor"=w1152:u32, "Frame thickness"=w1134:i32, "HeaderIcon"=w1138:u8[][])
        n538 = local read "_IconSize"() -> (w1129:u16)
        n539 = Unbundle By Name(w1135) -> ("BodyIcon"=w1158:u8[][])
        n540 = local read "_BodyBk"() -> (w1150:T2)
        n541 = Unbundle By Name(w1150) -> ("Color"=w1131:u32)
        n542 = Unbundle By Name(w1135) -> ("BgIcon"=w1159:u8[][], "BgIconOffset"=w1160:cluster{"X":i32, "Y":i32}, "BgIconMask"=w1162:u8[], "HeaderBkColor"=w1163:u32)
        n543 = Not Equal?(x=w1153, y=w1129) -> (x != y?=w1154:bool)
        n544 = call <resource>:"GDSLvIcon_Convert24bitTo8bitColor.vi"("Color 24bit In"=w1163) -> ("Color out(256)"=w1164:u8)  [unwired: 15 in, 3 out]
        n545 = call <resource>:"GDSLvIcon_Convert24bitTo8bitColor.vi"("Color 24bit In"=w1131) -> ("Color out(256)"=w1130:u8)  [unwired: 15 in, 3 out]
        n546 = Select(t=0, s=w1154, f=w1156) -> (s? t:f=w1157:i32)
        n547 = stacked-sequence {
          tunnel: w1149 -> [w1173]
          tunnel: [w1173] -> w1166
          tunnel: [w1172] -> w1169
          frame #0 {
            n548 = Tick Count (ms)() -> (millisecond timer value=w1172:u32)
          }
        }
        n549 = Build Array(w1164, w1130) -> (w1161:u8[])
        n550 = Unbundle By Name(w1135) -> ("ConnectorPaneHeight"=w1139:i32[], "BodyIconHeight"=w1140:i32)  [unwired: 1 out]
        n551 = Bundle By Name(cluster=w1146, "BgIcon"=w1159, "BgIconOffset"=w1160, "BgIconMask"=w1162, "ColorsOkayforiconToBeOnTopOf"=w1161) -> (w1165:T20)
        n552 = local read "_HideHeader"() -> (w1141:bool)
        n553 = call <resource>:"GDSIconEditor_IconSizeAdjustment.vi"("BodyIconHeightIn"=w1140, "HideHeader"=w1141, "ConnectorPaneHeight"=w1139, "Frame thickness"=w1134, "_IconSize"=w1129, "HeaderIconIn"=w1138) -> ("HeaderIconOut"=w1137:u8[][], "ImageRows"=w1136:i32)  [unwired: 3 in, 1 out]
        n554 = call <resource>:"GDSLvIcon_CreateIconPicture.vi"("FrameColor"=w1152, "FrameThickness(1)"=w1134, "HeaderIconIn"=w1137, "BodyIconIn"=w1158, "error in (no error)"=w1166, "ImageRows(32)"=w1136, "BigSizeIcon(x6)"=4, "RowStart(0)"=w1157, "BgIcon"=w1165) -> ("BodyIconOut"=w1133:u8[][], "WholeIconOut"=w1132:u8[][], "IconPictureOut"=w1143:picture, "LargeIconPictureOut(x6)"=w1142:picture, "error out"=w1167:errorcluster)  [unwired: 5 in, 1 out]
        n555 = case shown="\"UpdateIcon,Exit\"" w1145 {
          tunnel: ["Exit" ("item tag") "Idle" ("item tag")] -> w1147
          frame "UpdateIcon,Exit" {
          }
          frame Default {
          }
        }
        n556 = Bundle By Name(cluster=w1135, "CurrentIcon"=w1165, "RenameOption.IconOut"=w1133, "RenameOption.BgColor"=w1130) -> (w1144:T5)
        n557 = local write "_After"(w1143) -> ()
        n558 = stacked-sequence {
          tunnel: w1167 -> [w1171]
          tunnel: [w1171] -> w1148
          tunnel: [w1170] -> w1168
          tunnel: w1133 -> [_]
          tunnel: w1132 -> [_]
          frame #0 {
            n559 = Tick Count (ms)() -> (millisecond timer value=w1170:u32)
          }
        }
        n560 = local write "_IconPreview"(w1142) -> ()
        n561 = Subtract(x=w1168, y=w1169) -> ()  [unwired: 1 out]
      }
    }
    n562 = Equal?(x=w36, y="Exit") -> (x = y?=w39:bool)
    n563 = Select(t="Error", s=w35, f=w36) -> (s? t:f=w40:string)
  }
  "error out" <- w14
  n564 = Unbundle By Name(w16) -> ("Cancelled"=→"Cancelled":bool, "RenameOption"=→"RenameOption":T28)
  "ObjectOut" <- "ObjectIn"
